vi "Main_control_cRIO.vi"() -> ()   [LabVIEW 2022 SP3]
uses:
  <vilib>/Platform/TimedLoop/XDataNode/timing_clust.ctl
  <vilib>/Platform/TimedLoop/XDataNode/nitl_modes.ctl
  <vilib>/Platform/TimedLoop/XDataNode/wakeup.ctl
  <vilib>/Analysis/baseanly.llb/Mean (DBL).vi
  a7aeaaac-04ba-4589-9d9a-9c348744fe2e.vi
  <vilib>/FPGAPlugInAG/cRIO-9045/niLvFpga_Open_cRIO-9045.vi
  <vilib>/rvi/interface/common/dynamic/niFpgaDynamicAddResources.vi
  <vilib>/Modbus/slave/Create Slave Instance (TCP).vi
  <vilib>/Utility/error.llb/Error Cluster From Error Code.vi
  <vilib>/rvi/errors/niLvFpgaAdjustHostInterfaceError.vi
  <vilib>/FPGAPlugInAG/Dynamic/niLvFpga_Close_Dynamic.vi
  <vilib>/rvi/interface/nirviOpenFPGA/nirviOpenFPGA.xnode
  FPGA Bitfiles/crio_FPGATarget_FPGAcomp_QzR2OHjg63E.lvbitx
  FPGA_1.vi
  <vilib>/platform/TimedLoop/XDataNode/XDataNode.xnode
  <vilib>/Comparison/Less/Less Functor/Less Functor.lvclass
  <vilib>/rvi/interface/nirviReadWriteControl/nirviReadWriteControl.xnode
  <vilib>/rvi/interface/nirviCloseFPGA/nirviCloseFPGA.xnode
  <vilib>/Modbus/slave/Modbus Slave.lvclass
  <vilib>/Modbus/master/Modbus Master.lvclass
  <vilib>/Platform/TimedLoop/XDataNode/XDNodeRunTimeDep.lvlib
  SubVIs/DAQ/DAQ_Termopares.lvlib
  SubVIs/CC Modbus/CC_Library.lvlib
  <vilib>/Analysis/NI_AALBase.lvlib
  <vilib>/rvi/interface/Simulation/niFpgaSimulationCallBeginRW.vi
  NiFpgaLv.dll
  <vilib>/ptbypt/NI_PtbyPt.lvlib
panel:
  out "isCamChangingSet?":bool
  out "PID 6":u32
  out "PID 2":u32
  out "PID 4":u32
  out "PID 8":u32
  out "PID 7":u32
  out "PID 5":u32
  out "PID 1":u32
  out "PID 3":u32
  out "W1.13":bool
  out "1.15":bool
  out "W1.7":bool
  out "W1.9":bool
  out "W1.11":bool
  out "W1.5":bool
  out "W1.3":bool
  out "W1.1":bool
  out "Segmento act":u16
  in  "reset warnings":bool
  out "Warnings table out":T1(array[cluster]) {"Time Stamp" format="%<%.3X %x>T"}
  in  "Activar Sim Bitron":bool
  out "LEL":bool
  out "CO":bool
  out "O2":bool
  out "LEL (%)":dbl
  out "CO (%)":dbl
  out "O2 (%)":dbl
  out "Array Warnings":bool[](array[boolean])
  out "Guardando resumen":bool=TRUE
  out "path":path
  out "T estabilidad calor":u32
  out "T transitorio calor":u32
  out "T estabilidad frio":u32
  out "T transitorio frio":u32
  out "Timer 4 (Inicio Estabilidad Calor)":u32
  out "Timer 3 (Inicio Transitorio Calor)":u32
  in  "Configuración":T2(tab)
  in  "Setpoint calor cam":dbl=55.0
  in  "Setpoints peltiers":dbl=85.0
  in  "Setpoint calor corte rampa":dbl=51.0
  in  "Setpoint Frío":dbl=-40.0 min=-28.0 max=70.0 step=0.1
  in  "Setpoint Corte Frío":dbl=-30.0 min=-28.0 max=70.0 step=0.1
  in  "Tiempò en estabilidad de Frío":u32=15
  in  "Tiempo minimo de ciclo":u32=70
  in  "Tiempo maximo de ciclo":u32=90
  in  "Cam ºC/min":dbl=2.2
  in  "Pelt ºC/min":dbl=2.5
  in  "T cliclo (Bitron FSM Sim)":u32
  in  "FSM Bitron Simulacion":i32
  in  "EnablePIs":bool[](array[boolean])=[FALSE, FALSE, FALSE, TRUE, FALSE, TRUE, FALSE, FALSE]
  in  "descarte media":i32=1
  out "DO H2 LAB":bool
  out "Array":dbl[][](array[numeric])
  out "error out":errorcluster
  in  "Enable Test PID":bool
  in  "Disable PID":bool
  in  "Test PID":u32[](array[numeric])
  out "PWM array":u32[](array[numeric])
  out "T_valves":dbl[](array[numeric]) format="%0.2f"
  out "PWM 8 (%)":u32
  out "PWM 7 (%)":u32
  out "PWM 6 (%)":u32
  out "PWM 5 (%)":u32
  out "PWM 4 (%)":u32
  out "PWM 3 (%)":u32=50 max=100
  out "SGL values":dbl[](array[numeric])
  out "Int values":u16[](array[numeric])
  out "Guardando en disco":bool
  out "array w/ subset deleted":dbl[][](array[numeric])
  out "Guardar Array":dbl[][](array[numeric])
  out "size(s)":i32
  out "TCP Connection Count":u32
  out "mean_T_valves":dbl format="%0.2f"
  out "Holding registers":u16[](array[numeric])
  out "First Time":bool=TRUE
  out "Timer 1 (Inicio transitorio frio)":u32
  out "Timer 2 (Inicio Estabilidad Frio)":u32
  in  "Rampa_cam":bool
  out "Temp_valves":dbl[](array[numeric]) format="%0.2f"
  in  "Rampa_pelt":bool
  in  "Minutos de medio ciclo":dbl=70.0
  out "Minutos":dbl
  out "Ciclos Totales":dbl
  out "segundos":dbl
  out "días":dbl
  out "Horas":dbl
  out "Minutos Totales":dbl
  out "t ensayo (s)":u64
  in  "Reset tempo":bool
  out "Iteration Duration":i64
  in  "Desconex_Control_Hum":bool
  out "PWM 2 (%)":u32
  out "Program running":bool
  in  "Pausa entrar":bool
  in  "Segmento":u16
  in  "Pausa":bool
  in  "stop Control General":bool
  in  "Run Program":bool
  in  "Entrada digital Bitron":bool
  in  "Cam_Hum_write":dbl min=0.0 max=100.0 step=0.1
  in  "Cam_Write_Set_Hum":bool
  in  "Cam_Temp_write":dbl min=-28.0 max=70.0 step=0.1
  in  "Cam_Write_Set_Temp":bool
  out "Cam_Temp_read":dbl min=-28.0 max=70.0 step=0.1
  out "Cam_Hum_read":dbl min=-28.0 max=70.0 step=0.1
  in  "Setpoint Peltiers":dbl=25.0
  in  "enable_PI":bool
  out "PWM 1 (%)":u32=50 max=100
  in  "STOP ALL":bool
  # "Temporizadores de ciclo"
  # "PID1 TEST"
  # "PID2 TEST"
  # "PID3 TEST"
  # "PID4 TEST"
  # "PID5 TEST"
  # "PID6 TEST"
  # "PID7 TEST"
  # "PID8 TEST"
  # "Peltiers"
  # "Cámara climática"
  # "min"
  # "min"
  # "min"
  # "min"
  # "segmento"
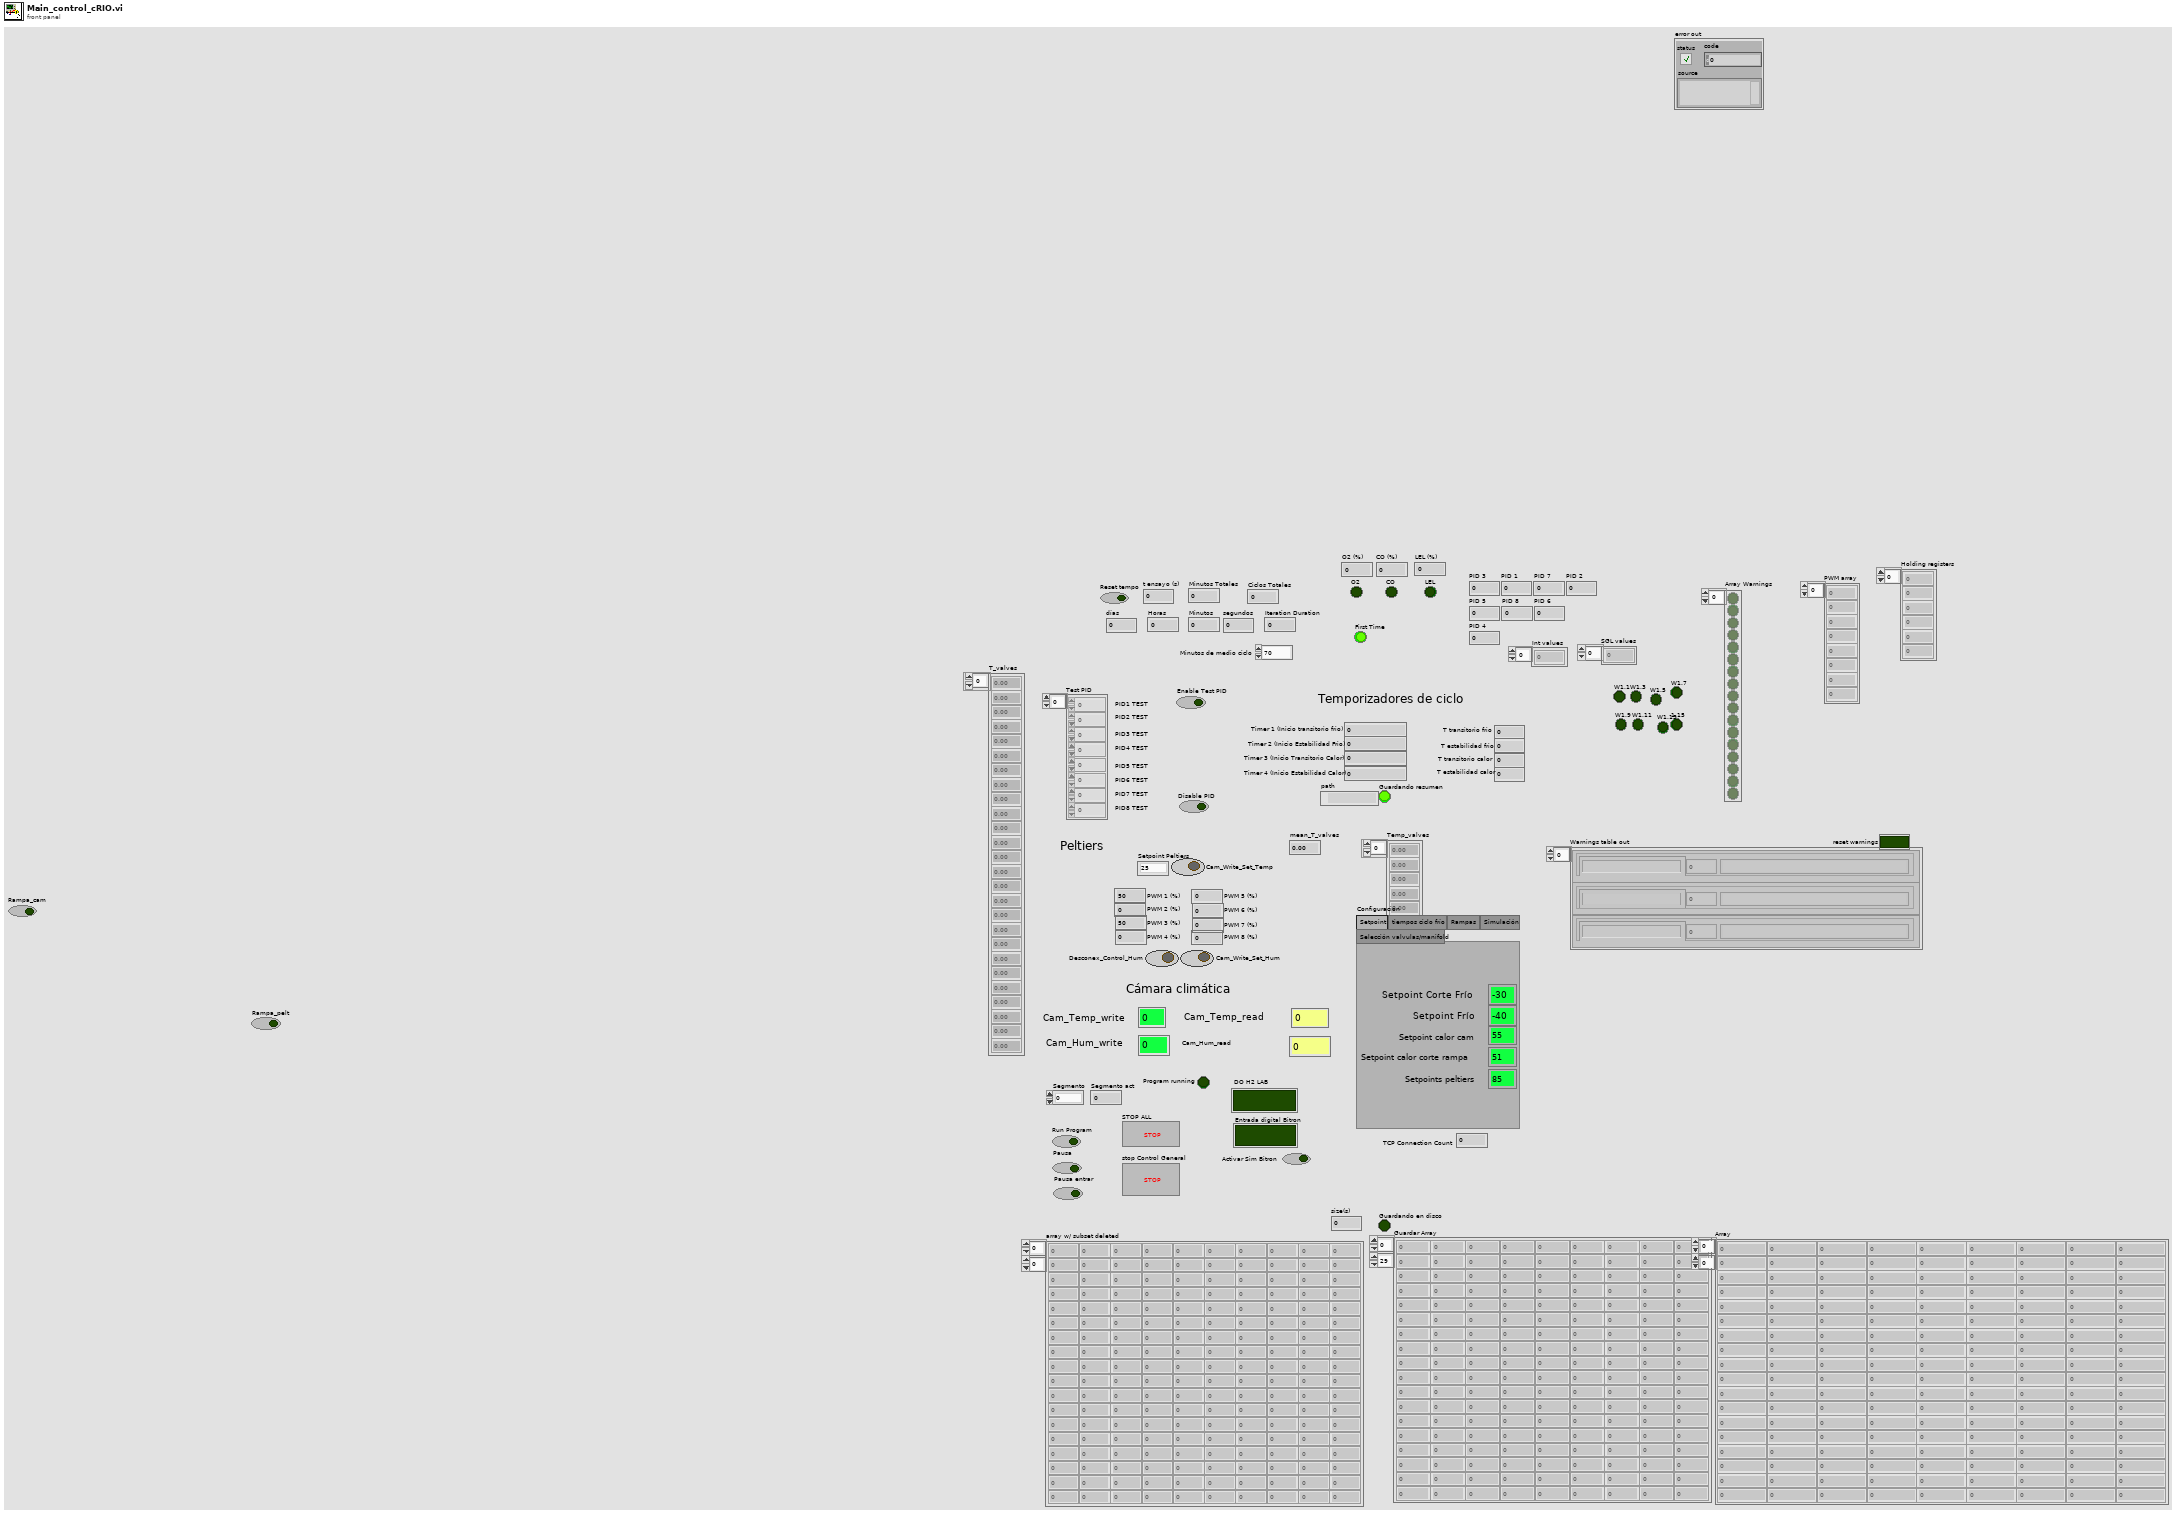
[diagram p1: front panel]
types:
  T1 = cluster{"Time Stamp":timestamp, "Descripcion":string, "Numeric":i32}[]
  T2 = enum32{"Setpoint", "tiempos ciclo frío", "Rampas ", "Simulación", "Selección valvulas/manifold"}
  T3 = enum8{"Enabled", "Disabled", "Disabled and Grayed Out"}
  T4 = typedef "XDNodeRunTimeDep.lvlib/timing_clust.ctl" = cluster{"Expected End [f-1]":u64, "Actual End [f-1]":u64, "Finished Late? [f-1]":bool, "Expected End [i-1]":u64, "Actual End [i-1]":u64, "Finished Late? [i-1]":bool, "Expected Start [i]":u64, "Actual Start [i]":u64, "Expected Start [f]":u64, "Actual Start [f]":u64, "Source Name":string, "Structure Name":string, "Period":i64, "Deadline":i64, "Offset":i64, "Start":i64, "Priority":i32, "Timeout":i32, "Mode":T5, "Wakeup Reason":T6, "Error":errorcluster, "Source Type":string, "Secondary Source Type":string, "Global End Time":u64, "Global Start Time":u64, "Frame Duration":u64, "Iteration Duration":u64, "Assigned CPU":i32, "I/O Scan Engine Mode":u32}
  T5 = typedef "XDNodeRunTimeDep.lvlib/nitl_modes.ctl" = enum32{"No Change", "Process missed periods, maintain original phase", "Discard missed periods, maintain original phase", "Process missed periods, ignore original phase", "Discard missed periods, ignore original phase"}
  T6 = typedef "XDNodeRunTimeDep.lvlib/wakeup.ctl" = enum32{"Normal", "Aborted", "Asynchronous wakeup", "Timing source error", "Timed loop error", "Timeout"}
  T7 = enum16{"open", "open or create", "create or replace", "create", "open (read-only)"}
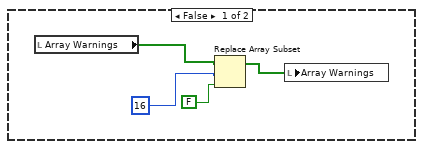
[diagram p3: hidden frame]
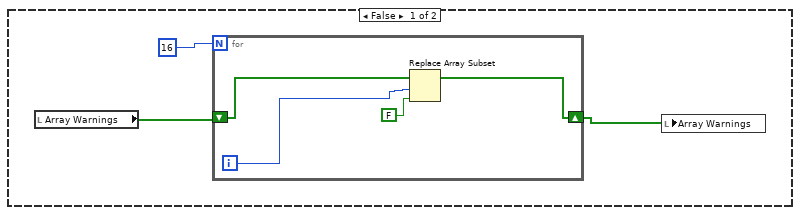
[diagram p4: hidden frame]
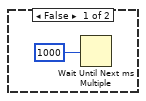
[diagram p7: hidden frame]
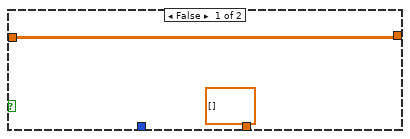
[diagram p8: hidden frame]
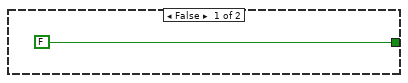
[diagram p9: hidden frame]
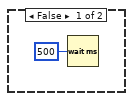
[diagram p14: hidden frame]
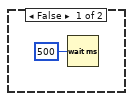
[diagram p15: hidden frame]
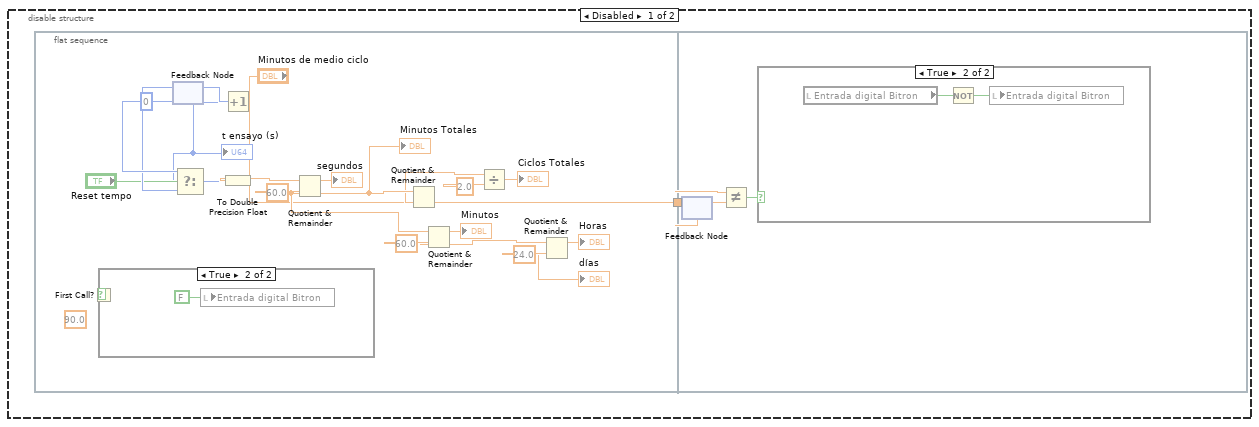
[diagram p17: hidden frame]
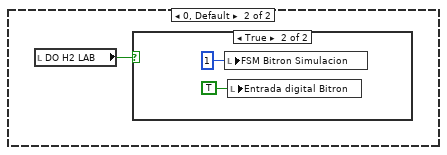
[diagram p20: hidden frame]
diagram:
  n1 = flat-sequence {
    tunnel: [w20] -> w16
    tunnel: [w19] -> w13
    tunnel: [w24] -> w12
    tunnel: [w29] -> w9
    tunnel: [w28] -> w8
    tunnel: [w22] -> w5
    tunnel: [w21] -> w4
    tunnel: [w17] -> w1
    tunnel: w16 -> [w61]
    tunnel: [w60] -> w15
    tunnel: [w59] -> w14
    tunnel: w13 -> [w58]
    tunnel: w12 -> [_]
    tunnel: [w51] -> w11
    tunnel: [w50] -> w10
    tunnel: w9 -> [w47]
    tunnel: w8 -> [w46]
    tunnel: [w45] -> w7
    tunnel: [w44] -> w6
    tunnel: w5 -> [_]
    tunnel: w4 -> [_]
    tunnel: [w32] -> w3
    tunnel: [w33] -> w2
    tunnel: w1 -> [_]
    tunnel: w15 -> [w1037]
    tunnel: w14 -> [w1036]
    tunnel: w11 -> [w1045]
    tunnel: w10 -> [w1044]
    tunnel: w7 -> [w1040]
    tunnel: w6 -> [w1039]
    tunnel: w3 -> [w1031]
    tunnel: w2 -> [w1032]
    frame #0 {
      w17 = FALSE ("Visible")
      w21 = bool[] [FALSE, FALSE, FALSE, FALSE, FALSE, FALSE, FALSE, FALSE, FALSE, FALSE, FALSE, FALSE, FALSE, FALSE, FALSE, FALSE, FALSE, FALSE, FALSE] ("Array Warnings")
      w22 = FALSE ("DO H2 LAB")
      w18 = u32 0 ("PWM 1 (%)")
      w26 = TRUE ("Visible")
      w30 = 10086 items=["J"=10072, "K"=10073, "N"=10077, "R"=10082, "S"=10085, "T"=10086, "B"=10047, "E"=10055] ("thermocouple type")
      w24 = FALSE ("Visible")
      n2 = local write "Entrada digital Bitron"(FALSE ("Entrada digital Bitron")) -> ()
      n3 = call "DAQ_connect.vi"("thermocouple type"=w30, "Array"=tag[] ["Mod2/ai0", "Mod2/ai1", "Mod2/ai2", "Mod2/ai3", "Mod2/ai4", "Mod2/ai5", "Mod2/ai6", "Mod2/ai7", "Mod2/ai8", "Mod2/ai9", "Mod2/ai10", "Mod2/ai11", "Mod2/ai12", "Mod2/ai13", "Mod2/ai14", "Mod2/ai15"]) -> ("error out"=w28:errorcluster, "Refnum out"=w29:refnum<k21>)  [unwired: 8 in]
      "error out" <- w28
      n4 = xnode "Open FPGA VI Reference"() -> ("FPGA VI Reference Out"=w20:refnum<k20>, "error out"=w19:errorcluster)  [unwired: 2 in]
      n5 = property on="Cam_Write_Set_Temp" class="Bool (strict)"("Visible"=w26) -> ()  [unwired: 2 in, 2 out]
      n6 = local write "PWM 8 (%)"(w18) -> ()
      n7 = property on="Cam_Write_Set_Hum" class="Bool (strict)"("Visible"=w26) -> ()  [unwired: 2 in, 2 out]
      n8 = local write "PWM 6 (%)"(w18) -> ()
      n9 = local write "PWM 7 (%)"(w18) -> ()
      n10 = local write "PWM 5 (%)"(w18) -> ()
      n11 = local write "PWM 4 (%)"(w18) -> ()
      n12 = local write "PWM 1 (%)"(w18) -> ()
      n13 = local write "PWM 2 (%)"(w18) -> ()
      n14 = local write "Rampa_pelt"(w24) -> ()
      n15 = local write "PWM 3 (%)"(w18) -> ()
      n16 = property on="enable_PI" class="Bool (strict)"("Visible"=w24) -> ()  [unwired: 2 in, 2 out]
      n17 = property on="Disable PID" class="Bool (strict)"("DisabledEnum"=T3."Disabled" ("Disabled")) -> ()  [unwired: 2 in, 2 out]
      n18 = local write "PID 8"(w18) -> ()
      n19 = local write "PID 7"(w18) -> ()
      n20 = local write "PID 6"(w18) -> ()
      n21 = local write "PID 5"(w18) -> ()
      n22 = local write "PID 1"(w18) -> ()
      n23 = local write "PID 2"(w18) -> ()
      n24 = local write "PID 4"(w18) -> ()
      n25 = local write "PID 3"(w18) -> ()
      n26 = property on="isCamChangingSet?" class="Bool (strict)"("Visible"=w17) -> ()  [unwired: 2 in, 2 out]
      "DO H2 LAB" <- w22
      "Array Warnings" <- w21
    }
    frame #1 {
      # "Running"
      n27 = node-c288() -> (w39:T4)  [unwired: 4 in]
      n28 = call "Nanodac_connect.vi"() -> ("error out"=w34:errorcluster, "Modbus Master out"=w35:refnum<class "Modbus Master.lvclass">)  [unwired: 10 in]
      n29 = node-c288() -> (w37:T4)  [unwired: 4 in]
      n30 = while "Adquisicion Resumen Datos/ciclo" {
        stop <- w237 stop-if-true
        w238 = FALSE ("Guardando resumen")
        # "CUIDADO! Al volver a empezar el ciclo, el Timer 1 va a ser el del siguiente ciclo, no el del que queremos registrar"
        # "0 -> First Time. Frío hasta -30 y señal bitron\n1 -> Transitorio frio\n2 -> Estabilidad frio\n3 -> Transitorio calor\n4 -> Estabilidad calor"
        # "Datos a guardar por ciclo:\n- Tiempo semiciclo frio\n- Tiempo estabilidad frio\n- Tiempo semiciclo calor\n- Tiempo estabilidad calor"
        n31 = local read "Segmento"() -> (w249:u16)
        n32 = feedback-in #1(w249) -> ()
        n33 = feedback #1(w249) -> (w248:u16)
        n34 = Equal?(x=w249, y=u16 1) -> (x = y?=w246:bool)
        n35 = local read "Program running"() -> (w235:bool)
        n36 = local write "Guardando resumen"(w238) -> ()
        n37 = local read "Segmento"() -> (w240:u16)
        n38 = Not Equal?(x=w248, y=u16 1) -> (x != y?=w245:bool)
        n39 = And(x=w246, y=w245) -> (x .and. y?=w236:bool)
        n40 = And(x=w235, y=w236) -> (x .and. y?=w234:bool)
        n41 = feedback #2(w240) -> (w241:u16)
        n42 = feedback-in #2(w240) -> ()
        n43 = Equal?(x=w240, y=u16 4) -> (x = y?=w243:bool)
        n44 = local read "Program running"() -> (w231:bool)
        n45 = case shown="True" w234 {
          tunnel: w238 -> [_ _]
          frame False {
          }
          frame True {
            n46 = flat-sequence {
              frame #0 {
                n47 = local read "Timer 4 (Inicio Estabilidad Calor)"() -> (w255:u32)
                n48 = local read "Timer 3 (Inicio Transitorio Calor)"() -> (w257:u32)
                n49 = local read "Timer 2 (Inicio Estabilidad Frio)"() -> (w258:u32)
                n50 = local read "Timer 1 (Inicio transitorio frio)"() -> (w256:u32)
                n51 = Subtract(x=w256, y=w255) -> (x-y=→"T estabilidad calor":u32)
                n52 = Subtract(x=w255, y=w257) -> (x-y=→"T transitorio calor":u32)
                n53 = Subtract(x=w257, y=w258) -> (x-y=→"T estabilidad frio":u32)
              }
              frame #1 {
                n54 = while {
                  stop <- w262 stop-if-true
                  n55 = local read "Guardando en disco"() -> (w263:bool)
                  n56 = Not(x=w263) -> (.not. x?=w262:bool)
                  n57 = Wait (ms)(milliseconds to wait=u32 500) -> ()  [unwired: 1 out]
                }
              }
              frame #2 {
                n58 = local read "T estabilidad calor"() -> (w268:u32)
                n59 = local read "T transitorio calor"() -> (w269:u32)
                n60 = local read "T estabilidad frio"() -> (w270:u32)
                n61 = local read "T transitorio frio"() -> (w271:u32)
                n62 = local read "path"() -> (w266:path)
                n63 = TDMS Open(10:T7."open or create" ("operation (0:open)"), 11:w266) -> (0:w276:errorcluster, 3:w277:refnum<k34>)  [unwired: 5 in]
                n64 = Build Array(w271, w270, w269, w268) -> (w267:u32[])
                n65 = TDMS Write(0:w277, 5:"Resumen Ciclos" ("group name in (Untitled)"), 7:string[] ["Time Transitorio frio (s)", "Time estabilidad frio (s)", "Time Transitorio calor (s)", "Time estabilidad calor (s)"] ("channel name(s) in (Untitled)"), 9:w267, 11:w276) -> (4:w275:refnum<k34>, 15:w274:errorcluster)  [unwired: 1 in, 2 out]
                n66 = TDMS Close(8:w274, 11:w275) -> ()  [unwired: 2 out]
                "Guardando resumen" <- TRUE
              }
            }
          }
        }
        n67 = Not Equal?(x=w241, y=u16 4) -> (x != y?=w244:bool)
        n68 = And(x=w243, y=w244) -> (x .and. y?=w233:bool)
        n69 = And(x=w233, y=w231) -> (x .and. y?=w232:bool)
        n70 = case shown="True" w232 {
          frame False {
          }
          frame True {
            n71 = local read "Timer 1 (Inicio transitorio frio)"() -> (w252:u32)
            n72 = local read "Timer 2 (Inicio Estabilidad Frio)"() -> (w251:u32)
            n73 = Subtract(x=w251, y=w252) -> (x-y=→"T transitorio frio":u32)
          }
        }
        n74 = local read "STOP ALL"() -> (w237:bool)
        n75 = Wait (ms)(milliseconds to wait=u32 500) -> ()  [unwired: 1 out]
      }
      n76 = timed-loop "Rampa SP Camara" {
        timing: w39 -> [_]
        timing-out: [_] -> w38
        stop <- w592 stop-if-true
        n77 = node-c288() -> ()  [unwired: 1 in, 1 out]
        n78 = case shown="True" "Rampa_cam" {
          frame False {
            n79 = Wait (ms)(milliseconds to wait=u32 500) -> ()  [unwired: 1 out]
          }
          frame True {
            n80 = flat-sequence {
              tunnel: [w602] -> w594
              tunnel: w594 -> [w617]
              frame #0 {
                # "10*1/3*10^-4 ºC cada 20ms"
                n81 = local read "Cam_Temp_write"() -> (w608:dbl)
                n82 = local read "Temp_valves"() -> (w600:dbl[])
                n83 = Divide(x=1.0, y=3.0) -> (x/y=w614:dbl)
                n84 = Multiply(x="Cam ºC/min", y=w614) -> (x*y=w612:dbl)
                n85 = Index Array(array=w600, index #1=0 ("index"), index #2=1 ("index")) -> (element #1=w597:dbl, element #2=w596:dbl)
                n86 = Divide(x=w612, y=1000.0) -> (x/y=w613:dbl)
                n87 = Add(x=w608, y=w613) -> (x+y=w610:dbl)
                n88 = Build Array(w597, w596) -> (w595:dbl[])
                n89 = call-poly <vilib>:"Mean.vi"("X"=w595) -> ("mean"=w601:dbl)  [unwired: 1 out]
                n90 = Greater Or Equal?(x=w610, y="Setpoint calor cam") -> (x >= y?=w603:bool)
                n91 = Greater Or Equal?(x=w601, y="Setpoint calor corte rampa") -> (x >= y?=w604:bool)
                n92 = Or(x=w603, y=w604) -> (x .or. y?=w602:bool)
                n93 = Select(t="Setpoint calor cam", s=w602, f=w610) -> (s? t:f=w609:dbl)
                n94 = local write "Cam_Temp_write"(w609) -> ()
              }
              frame #1 {
                n95 = Not(x=w617) -> (.not. x?=w618:bool)
                n96 = local write "Rampa_cam"(w618) -> ()
              }
            }
          }
        }
        n97 = local read "STOP ALL"() -> (w592:bool)
        n98 = node-c288() -> ()  [unwired: 1 in, 1 out]
      }
      n99 = node-c288() -> (w63:T4)  [unwired: 4 in]
      n100 = timed-loop "Warnings/Errores" {
        timing: w37 -> [_]
        timing-out: [_] -> w36
        shift-right: [w78] -> _
        shift-left: T1 [] ("Warnings table out") -> [w79]
        stop <- w81 stop-if-true
        n101 = node-c288() -> ()  [unwired: 1 in, 1 out]
        n102 = local read "Program running"() -> (w84:bool)
        n103 = local read "Pausa"() -> (w85:bool)
        n104 = Not(x=w85) -> (.not. x?=w83:bool)
        n105 = And(x=w84, y=w83) -> (x .and. y?=w82:bool)
        n106 = case shown="True" w82 {
          frame False {
          }
          frame True {
            # "0 -> First Time. Frío hasta -30 y señal bitron\n1 -> Transitorio frio\n2 -> Estabilidad frio\n3 -> Transitorio calor\n4 -> Estabilidad calor"
            # "Si estamos en semiciclo de calor\ny no hay pausa"
            n107 = local read "Segmento"() -> (w137:u16)
            n108 = Tick Count (ms)() -> (millisecond timer value=w131:u32)
            n109 = local read "LEL (%)"() -> (w124:dbl)
            n110 = feedback-in #3(w131) -> ()
            n111 = feedback #3(w131) -> (w130:u32)
            n112 = local read "Array Warnings"() -> (w120:bool[])
            n113 = local read "isCamChangingSet?"() -> (w89:bool)
            n114 = Equal?(x=w137, y=u16 3) -> (x = y?=w134:bool)
            n115 = Equal?(x=w137, y=u16 4) -> (x = y?=w133:bool)
            n116 = Subtract(x=w131, y=w130) -> (x-y=w129:u32)
            n117 = Greater?(x=w124, y=3.0) -> (0:w118:bool)
            n118 = Or(x=w134, y=w133) -> (x .or. y?=w132:bool)
            n119 = Replace Array Subset(array=w120, new element=w118, index=17) -> (w117:bool[])
            n120 = Select(t=u32 1000, s=w89, f=u32 60000 ("y")) -> (s? t:f=w86:u32)
            n121 = Greater Or Equal?(x=w129, y=w86) -> (x >= y?=w128:bool)
            n122 = Array Subset(array=w117, index=0, length=19) -> (w110:bool[])
            n123 = case shown="True" w132 {
              frame False {
                n124 = local read "Array Warnings"() -> (w169:bool[])
                n125 = for {
                  N: 16 -> [_]
                  shift-right: [w171] -> w168
                  shift-left: w169 -> [w172]
                  i -> [w174]
                  n126 = Replace Array Subset(array=w172, new element=FALSE ("new element/subarray"), index=w174) -> (w171:bool[])
                }
                n127 = local write "Array Warnings"(w168) -> ()
              }
              frame True {
                n128 = local read "Setpoint Peltiers"() -> (w215:dbl)
                n129 = local read "T_valves"() -> (w214:dbl[])
                n130 = for {
                  N: 16 -> [_]
                  tunnel: w215 -> [w222]
                  tunnel: w214 -> [w220]
                  shift-right: [w216] -> w195
                  shift-left: bool[] [FALSE, FALSE, FALSE, FALSE, FALSE, FALSE, FALSE, FALSE, FALSE, FALSE, FALSE, FALSE, FALSE, FALSE, FALSE, FALSE] -> [w217]
                  i -> [w219]
                  n131 = Index Array(array=w220, index=w219) -> (element=w218:dbl)
                  n132 = Subtract(x=w222, y=w218) -> (x-y=w225:dbl)
                  n133 = Absolute Value(x=w225) -> (abs(x)=w224:dbl)
                  n134 = Greater?(x=w224, y=20.0) -> (0:w221:bool)
                  n135 = Replace Array Subset(array=w217, new element=w221, index=w219) -> (w216:bool[])
                }
                n136 = local read "Array Warnings"() -> (w194:bool[])
                n137 = Index Array(array=w195, index #1=0 ("index"), index #2=2 ("index"), index #3=4 ("index"), index #4=6 ("index"), index #5=8 ("index"), index #6=10 ("index"), index #7=12 ("index"), index #8=14 ("index"), index #9=1 ("index"), index #10=3 ("index"), index #11=5 ("index"), index #12=7 ("index"), index #13=9 ("index"), index #14=11 ("index"), index #15=13 ("index"), index #16=15 ("index")) -> (element #1=w211:bool, element #2=w210:bool, element #3=w209:bool, element #4=w208:bool, element #5=w207:bool, element #6=w206:bool, element #7=w205:bool, element #8=w204:bool, element #9=w203:bool, element #10=w202:bool, element #11=w201:bool, element #12=w200:bool, element #13=w199:bool, element #14=w198:bool, element #15=w197:bool, element #16=w196:bool)
                n138 = Build Array(w211, w210, w209, w208, w207, w206, w205, w204, w203, w202, w201, w200, w199, w198, w197, w196) -> (w192:bool[])
                n139 = Replace Array Subset(array=w194, new element=w192, index=0) -> (w191:bool[])
                n140 = local write "Array Warnings"(w191) -> ()
              }
            }
            n141 = case shown="True" w128 {
              tunnel: w129 -> [_ w164]
              frame False {
                n142 = local read "Array Warnings"() -> (w141:bool[])
                n143 = Replace Array Subset(array=w141, new element=FALSE ("new element/subarray"), index=16) -> (w138:bool[])
                n144 = local write "Array Warnings"(w138) -> ()
              }
              frame True {
                n145 = local read "Cam_Temp_write"() -> (w155:dbl)
                n146 = local read "Cam_Temp_read"() -> (w153:dbl)
                n147 = Subtract(x=w153, y=w155) -> (x-y=w167:dbl)
                n148 = feedback #4(w153) -> (w154:dbl)
                n149 = feedback-in #4(w153) -> ()
                n150 = Absolute Value(x=w167) -> (abs(x)=w145:dbl)
                n151 = Subtract(x=w153, y=w154) -> (x-y=w165:dbl)
                n152 = Greater Or Equal?(x=w145, y=3.0) -> (x >= y?=w144:bool)
                n153 = Absolute Value(x=w165) -> (abs(x)=w161:dbl)
                n154 = Divide(x=w164, y=u32 60000) -> (x/y=w162:dbl)
                n155 = Divide(x=w161, y=w162) -> (x/y=w148:dbl)
                n156 = call <vilib>:"Mean PtByPt.vi"("x"=w148) -> ("mean"=w147:dbl)  [unwired: 3 in, 1 out]
                n157 = feedback-in #5(w145) -> ()
                n158 = feedback #5(w145) -> (w146:dbl)
                n159 = Not Equal To 0?(x=w146) -> (x != 0?=w142:bool)
                "isCamChangingSet?" <- w142
                n160 = Less?(x=w147, y=0.2) -> (x < y?=w159:bool)
                n161 = And(x=w142, y=w144) -> (x .and. y?=w143:bool)
                n162 = local read "Array Warnings"() -> (w150:bool[])
                n163 = First Call?() -> (First Call?: T/F=w156:bool)
                n164 = And(x=w143, y=w159) -> (x .and. y?=w158:bool)
                n165 = Not(x=w156) -> (.not. x?=w157:bool)
                n166 = And(x=w157, y=w158) -> (x .and. y?=w149:bool)
                n167 = Replace Array Subset(array=w150, new element=w149, index=16) -> (w152:bool[])
                n168 = local write "Array Warnings"(w152) -> ()
              }
            }
            n169 = local write "Array Warnings"(w110) -> ()
            n170 = local read "O2 (%)"() -> (w109:dbl)
            n171 = local read "Array Warnings"() -> (w123:bool[])
            n172 = Greater?(x=w109, y=25.0) -> (0:w125:bool)
            n173 = Less?(x=w109, y=10.0) -> (x < y?=w107:bool)
            n174 = Or(x=w125, y=w107) -> (x .or. y?=w121:bool)
            n175 = Replace Array Subset(array=w123, new element=w121, index=18) -> (w112:bool[])
            n176 = Array Subset(array=w112, index=0, length=19) -> (w111:bool[])
            n177 = local write "Array Warnings"(w111) -> ()
            n178 = local read "Array Warnings"() -> (w106:bool[])
            n179 = Index Array(array=w106, index #1=0 ("index"), index #2=2 ("index"), index #3=4 ("index"), index #4=6 ("index"), index #5=8 ("index"), index #6=10 ("index"), index #7=12 ("index"), index #8=14 ("index")) -> (element #1=→"W1.1":bool, element #2=→"W1.3":bool, element #3=→"W1.5":bool, element #4=→"W1.7":bool, element #5=→"W1.9":bool, element #6=→"W1.11":bool, element #7=→"W1.13":bool, element #8=→"1.15":bool)
          }
        }
        n180 = local read "Array Warnings"() -> (w80:bool[])
        n181 = call "Historical Warnings (SubVI).vi"("Warnings bool array"=w80, "in"="reset warnings", "warnings table in"=w79) -> ("Warnings table out"=w78:T1)  [unwired: 8 in]
        "Warnings table out" <- w78
        n182 = local read "STOP ALL"() -> (w81:bool)
        n183 = node-c288() -> ()  [unwired: 1 in, 1 out]
      }
      n184 = while "MODBUS CC NANODAC" {
        tunnel: w35 -> [w76]
        tunnel: w34 -> [w75]
        tunnel: [w65] -> w33
        tunnel: [w64] -> w32
        stop <- w74 stop-if-true
        n185 = call "Nanodac_lectura.vi"("Modbus Master in"=w76, "error in (no error)"=w75) -> ("Modbus Master out"=w65:refnum<class "Modbus Master.lvclass">, 16:"O2, CO, LEL"=w72:dbl[], 17:"O2, CO, LEL"=w73:bool[], "error out"=w64:errorcluster)  [unwired: 14 in]
        n186 = Index Array(array=w73) -> (element #1=→"O2":bool, element #2=→"CO":bool, element #3=→"LEL":bool)  [unwired: 3 in]
        n187 = Index Array(array=w72) -> (element #1=→"O2 (%)":dbl, element #2=→"CO (%)":dbl, element #3=→"LEL (%)":dbl)  [unwired: 3 in]
        n188 = local read "STOP ALL"() -> (w74:bool)
      }
      n189 = while "Modbus Slave" {
        stop <- w405 stop-if-true
        n190 = call-poly <vilib>:"Create Slave Instance.vi"() -> ("error out"=w408:errorcluster, "TCP slave instance"=w409:refnum<class "Modbus Slave.lvclass">)  [unwired: 10 in]
        n191 = while {
          shift-right: [w421] -> w407
          shift-left: w409 -> [w423]
          shift-right: [w420] -> w406
          shift-left: w408 -> [w422]
          stop <- w415 stop-if-true
          n192 = property class="Modbus Slave"(reference=w423, error in=w422) -> (reference out=w421:refnum<class "Modbus Slave.lvclass">, error out=w420:errorcluster, "Data Access:TCP Connection Count"=w419:u32)
          "TCP Connection Count" <- w419
          n193 = Not Equal?(x=w419, y=u32 0) -> (x != y?=w417:bool)
          n194 = local read "STOP ALL"() -> (w416:bool)
          n195 = Or(x=w417, y=w416) -> (x .or. y?=w415:bool)
        }
        n196 = node-c288() -> (w414:T4)  [unwired: 4 in]
        n197 = timed-loop {
          timing: w414 -> [_]
          timing-out: [_] -> w413
          shift-right: [w488] -> w411
          shift-left: w407 -> [w499]
          shift-right: [w487] -> w410
          shift-left: w406 -> [w497]
          shift-right: [w490] -> _
          shift-left: u16[] [0, 0, 0, 0, 0, 0, 0, 0, 0, 0, 0, 0, 0, 0, 0, 0, 0, 0, 0, 0, 0, 0, 0, 0, 0, 0, 0, 0, 0, 0, 0, 0, 0, 0, 0, 0, 0, 0, 0, 0, 0, 0, 0, 0, 0] -> [w491]
          stop <- w483 stop-if-true
          # "Temp_BobV3-8"
          # "Temp_valves\nTemp_bobs"
          n198 = node-c288() -> ()  [unwired: 1 in, 1 out]
          n199 = local read "Entrada digital Bitron"() -> (w472:bool)
          n200 = local read "Array Warnings"() -> (w455:bool[])
          n201 = local read "Program running"() -> (w504:bool)
          n202 = local read "DO H2 LAB"() -> (w459:bool)
          n203 = local read "T_valves"() -> (w467:dbl[])
          n204 = local read "enable_PI"() -> (w503:bool)
          n205 = local read "Cam_Temp_write"() -> (w468:dbl)
          n206 = local read "Cam_Temp_read"() -> (w469:dbl)
          n207 = local read "Cam_Hum_read"() -> (w471:dbl)
          n208 = local read "Cam_Hum_write"() -> (w470:dbl)
          n209 = local read "mean_T_valves"() -> (w434:dbl)
          n210 = local read "Setpoint Peltiers"() -> (w502:dbl)
          n211 = Build Array (concatenate)(w504, w503, w472, w459, w455) -> (w498:bool[])
          n212 = Build Array(w471, w470, w469, w468, w434) -> (w465:dbl[])
          n213 = Build Array(w502) -> (w466:dbl[])
          n214 = local read "Segmento act"() -> (w501:u16)
          n215 = local read "PWM array"() -> (w461:u32[])
          n216 = Build Array (concatenate)(w466, w467, w465) -> (w464:dbl[])
          "SGL values" <- w464
          n217 = Array Size(array=w464) -> (size(s)=w492:i32)
          n218 = To Unsigned Word Integer(number=w461) -> (unsigned 16bit integer=w462:u16[])
          n219 = call-dynamic "Write Multiple Coils.vi"("error in (no error)"=w497, "coil values"=w498, "starting address"=u16 1, "Modbus slave in"=w499) -> ("error out"=w494:errorcluster, "Modbus slave out"=w495:refnum<class "Modbus Slave.lvclass">)  [unwired: 6 in]
          n220 = Build Array(w501) -> (w463:u16[])
          n221 = Build Array (concatenate)(w463, w462) -> (w460:u16[])
          "Int values" <- w460
          n222 = for {
            N: w492 -> [_]
            tunnel: w464 -> [w586] mode=indexing
            shift-right: [w577] -> w490
            shift-left: w491 -> [w578]
            i -> [w585]
            n223 = call "double_2u16.vi"("Entrada"=w586) -> ("Salida 2"=w582:u16, "Salida 1"=w583:u16)  [unwired: 9 in]
            n224 = Multiply(x=2, y=w585) -> (x*y=w581:i32)
            n225 = Add(x=1, y=w581) -> (x+y=w579:i32)
            n226 = Replace Array Subset(array=w578, new element #1=w583, index #1=w581, new element #2=w582, index #2=w579) -> (w577:u16[])
          }
          n227 = for {
            tunnel: w460 -> [w576] mode=indexing
            tunnel: [w574] -> w489 mode=indexing
            n228 = Add(x=w576, y=u16 10000) -> (x+y=w574:u16)
          }
          n229 = Build Array (concatenate)(w489, w490) -> (w493:u16[])
          "Holding registers" <- w493
          n230 = call-dynamic "Write Multiple Holding Registers.vi"("error in (no error)"=w494, "holding register values"=w493, "starting address"=u16 100, "Modbus slave in"=w495) -> ("error out"=w480:errorcluster, "Modbus slave out"=w481:refnum<class "Modbus Slave.lvclass">)  [unwired: 6 in]
          n231 = call-dynamic "Read Coils.vi"("error in (no error)"=w480, "number of coils"=u16 5, "starting address"=u16 200, "Modbus slave in"=w481) -> ("error out"=w457:errorcluster, "coil values"=w474:bool[], "Modbus slave out"=w458:refnum<class "Modbus Slave.lvclass">)  [unwired: 5 in]
          n232 = Index Array(array=w474) -> (element #1=w477:bool, element #2=w476:bool, element #3=w475:bool, element #4=w473:bool, element #5=w456:bool)  [unwired: 5 in]
          n233 = local write "Run Program"(w477) -> ()
          n234 = local write "Pausa"(w476) -> ()
          n235 = local write "Pausa entrar"(w475) -> ()
          n236 = local write "stop Control General"(w473) -> ()
          n237 = case shown="True" w456 {
            tunnel: [w532 w534] -> w433
            tunnel: w458 -> [w532 w542]
            tunnel: w457 -> [w531 w541]
            tunnel: [w531 w533] -> w432
            frame False {
            }
            frame True {
              w545 = u16 22 ("number of holding registers")
              n238 = call-dynamic "Read Coils.vi"("error in (no error)"=w541, "number of coils"=u16 1, "starting address"=u16 205, "Modbus slave in"=w542) -> ("error out"=w540:errorcluster, "coil values"=w535:bool[], "Modbus slave out"=w539:refnum<class "Modbus Slave.lvclass">)  [unwired: 5 in]
              n239 = Index Array(array=w535) -> (element=w536:bool)  [unwired: 1 in]
              n240 = local write "Activar Sim Bitron"(w536) -> ()
              n241 = Quotient & Remainder(x=w545, y=u16 2) -> (floor(x/y)=w543:u16)  [unwired: 1 out]
              n242 = call-dynamic "Read Holding Registers.vi"("error in (no error)"=w540, "number of holding registers"=w545, "starting address"=u16 300, "Modbus slave in"=w539) -> ("error out"=w533:errorcluster, "register values"=w558:u16[], "Modbus slave out"=w534:refnum<class "Modbus Slave.lvclass">)  [unwired: 5 in]
              n243 = for {
                N: w543 -> [_]
                tunnel: [w566] -> w557 mode=indexing
                tunnel: w558 -> [w562]
                i -> [w573]
                n244 = Multiply(x=2, y=w573) -> (x*y=w571:i32)
                n245 = Add(x=w571, y=1) -> (x+y=w569:i32)
                n246 = Index Array(array=w562, index #1=w571, index #2=w569) -> (element #1=w561:u16, element #2=w560:u16)
                n247 = Join Numbers(hi=w561, lo=w560) -> ((hi.lo)=w568:u32)
                n248 = To Single Precision Float(number=w568) -> (single precision float=w565:sgl)
                n249 = Subtract(x=w565, y=sgl 10000.0) -> (x-y=w563:sgl)
                n250 = Divide(x=w563, y=sgl 100.0) -> (x/y=w566:sgl)
              }
              n251 = Index Array(array=w557) -> (element #1=w556:sgl, element #2=w555:sgl, element #3=w554:sgl, element #4=w553:sgl, element #5=w552:sgl, element #6=w551:sgl, element #7=w550:sgl, element #8=w549:sgl, element #9=w548:sgl, element #10=w547:sgl, element #11=w546:sgl)  [unwired: 11 in]
              n252 = local write "Tiempò en estabilidad de Frío"(w551) -> ()
              n253 = local write "Setpoint calor corte rampa"(w553) -> ()
              n254 = local write "Tiempo maximo de ciclo"(w549) -> ()
              n255 = local write "Tiempo minimo de ciclo"(w550) -> ()
              n256 = local write "T cliclo (Bitron FSM Sim)"(w546) -> ()
              n257 = local write "Setpoint Corte Frío"(w556) -> ()
              n258 = local write "Setpoint calor cam"(w554) -> ()
              n259 = local write "Setpoints peltiers"(w552) -> ()
              n260 = local write "Setpoint Frío"(w555) -> ()
              n261 = local write "Cam ºC/min"(w548) -> ()
              n262 = local write "Pelt ºC/min"(w547) -> ()
            }
          }
          n263 = call-dynamic "Read Coils.vi"("error in (no error)"=w432, "number of coils"=u16 1, "starting address"=u16 400, "Modbus slave in"=w433) -> ("error out"=w428:errorcluster, "coil values"=w429:bool[], "Modbus slave out"=w427:refnum<class "Modbus Slave.lvclass">)  [unwired: 5 in]
          n264 = Index Array(array=w429) -> (element=w424:bool)  [unwired: 1 in]
          n265 = local write "Disable PID"(w424) -> ()
          n266 = case shown="True" w424 {
            tunnel: w428 -> [w505 w520]
            tunnel: w427 -> [w506 w521]
            tunnel: [w506 w508] -> w426
            tunnel: [w505 w507] -> w425
            frame False {
            }
            frame True {
              n267 = call-dynamic "Read Holding Registers.vi"("error in (no error)"=w520, "number of holding registers"=u16 8, "starting address"=u16 410, "Modbus slave in"=w521) -> ("error out"=w507:errorcluster, "register values"=w517:u16[], "Modbus slave out"=w508:refnum<class "Modbus Slave.lvclass">)  [unwired: 5 in]
              n268 = Index Array(array=w517) -> (element #1=w516:u16, element #2=w515:u16, element #3=w514:u16, element #4=w513:u16, element #5=w512:u16, element #6=w511:u16, element #7=w510:u16, element #8=w509:u16)  [unwired: 8 in]
              n269 = local write "PWM 4 (%)"(w513) -> ()
              n270 = local write "PWM 1 (%)"(w516) -> ()
              n271 = local write "PWM 2 (%)"(w515) -> ()
              n272 = local write "PWM 5 (%)"(w512) -> ()
              n273 = local write "PWM 6 (%)"(w511) -> ()
              n274 = local write "PWM 7 (%)"(w510) -> ()
              n275 = local write "PWM 8 (%)"(w509) -> ()
              n276 = local write "PWM 3 (%)"(w514) -> ()
            }
          }
          n277 = local read "STOP ALL"() -> (w482:bool)
          n278 = call-dynamic "Read Coils.vi"("error in (no error)"=w425, "number of coils"=u16 8, "starting address"=u16 240, "Modbus slave in"=w426) -> ("error out"=w435:errorcluster, "coil values"=w445:bool[], "Modbus slave out"=w436:refnum<class "Modbus Slave.lvclass">)  [unwired: 5 in]
          n279 = local write "EnablePIs"(w445) -> ()
          n280 = call-dynamic "Read Holding Registers.vi"("error in (no error)"=w435, "number of holding registers"=u16 1, "starting address"=u16 350, "Modbus slave in"=w436) -> ("error out"=w437:errorcluster, "register values"=w441:u16[], "Modbus slave out"=w438:refnum<class "Modbus Slave.lvclass">)  [unwired: 5 in]
          n281 = Index Array(array=w441) -> (element=w442:u16)  [unwired: 1 in]
          n282 = local write "descarte media"(w442) -> ()
          n283 = call-dynamic "Read Coils.vi"("error in (no error)"=w437, "number of coils"=u16 1, "starting address"=u16 250, "Modbus slave in"=w438) -> ("error out"=w451:errorcluster, "coil values"=w448:bool[], "Modbus slave out"=w452:refnum<class "Modbus Slave.lvclass">)  [unwired: 5 in]
          n284 = Index Array(array=w448, index=0) -> (element=w446:bool)
          n285 = local write "Enable Test PID"(w446) -> ()
          n286 = case shown="True" w446 {
            tunnel: [w523 w530] -> w454
            tunnel: [w522 w529] -> w453
            tunnel: w452 -> [w523 w528]
            tunnel: w451 -> [w522 w527]
            frame False {
            }
            frame True {
              n287 = call-dynamic "Read Holding Registers.vi"("error in (no error)"=w527, "number of holding registers"=u16 8, "starting address"=u16 260, "Modbus slave in"=w528) -> ("error out"=w529:errorcluster, "register values"=w524:u16[], "Modbus slave out"=w530:refnum<class "Modbus Slave.lvclass">)  [unwired: 5 in]
              n288 = local write "Test PID"(w524) -> ()
            }
          }
          n289 = property class="Modbus Slave"(reference=w454, error in=w453) -> (reference out=w488:refnum<class "Modbus Slave.lvclass">, error out=w487:errorcluster, "Data Access:TCP Connection Count"=w486:u32)
          n290 = Equal?(x=w486, y=u32 0) -> (x = y?=w484:bool)
          n291 = Or(x=w484, y=w482) -> (x .or. y?=w483:bool)
          n292 = node-c288() -> ()  [unwired: 1 in, 1 out]
        }
        n293 = node-c288(w413) -> ()  [unwired: 1 out]
        n294 = local read "STOP ALL"() -> (w405:bool)
        n295 = call-dynamic "Close.vi"("error in (no error)"=w410, "Modbus slave in"=w411) -> ()  [unwired: 9 in, 1 out]
      }
      n296 = timed-loop "FPGA Aquisicion y control" {
        timing: w63 -> [_]
        timing-out: [_] -> w62
        tunnel: w61 -> [w1016]
        tunnel: [w999] -> w60
        tunnel: [w1015] -> w59
        tunnel: w58 -> [w1014]
        tunnel: w47 -> [w1013]
        tunnel: w46 -> [w1012]
        tunnel: [w1011] -> w45
        tunnel: [w1010] -> w44
        stop <- "STOP ALL" stop-if-true
        # "1 y 1 de momento, cuando haya mas valvulas, 2 y 2"
        n297 = node-c288() -> ()  [unwired: 1 in, 1 out]
        n298 = local read "PWM 8 (%)"() -> (w1000:u32)
        n299 = local read "PWM 6 (%)"() -> (w1002:u32)
        n300 = local read "PWM 7 (%)"() -> (w1001:u32)
        n301 = local read "PWM 5 (%)"() -> (w1003:u32)
        n302 = local read "PWM 4 (%)"() -> (w1004:u32)
        n303 = local read "PWM 1 (%)"() -> (w1007:u32)
        n304 = local read "PWM 2 (%)"() -> (w1006:u32)
        n305 = local read "PWM 3 (%)"() -> (w1005:u32)
        n306 = xnode "Read/Write Control"("FPGA VI Reference In"=w1016, "error in"=w1014, "PWM_DO0"=w1007, "PWM_DO1"=w1006, "PWM_DO2"=w1005, "PWM_DO3"=w1004, "PWM_DO4"=w1003, "PWM_DO5"=w1002, "PWM_DO6"=w1001, "PWM_DO7"=w1000) -> ("FPGA VI Reference Out"=w999:refnum<k20>, "error out"=w1015:errorcluster)
        n307 = call "DAQ_read_T_dT.vi"("error in (no error)"=w1012, "Refnum in"=w1013) -> ("error out"=w1010:errorcluster, "data"=w986:dbl[], "Refnum out"=w1011:refnum<k21>)  [unwired: 7 in]
        "Temp_valves" <- w986
        "T_valves" <- w986
        n308 = Build Array(w1007, w1006, w1005, w1004, w1003, w1002, w1001, w1000) -> (→"PWM array":u32[])
        n309 = local read "EnablePIs"() -> (w998:bool[])
        n310 = Split 1D Array(array=w986, index=8) -> (second subarray=w996:dbl[])  [unwired: 1 out]
        n311 = for {
          tunnel: w998 -> [w1018] mode=indexing
          tunnel: w996 -> [w1021] mode=indexing
          shift-right: [w1019] -> w995
          shift-left: dbl[] [] -> [w1020]
          n312 = case shown="False" w1018 {
            tunnel: w1021 -> [_ w1025]
            tunnel: w1020 -> [w1022 w1024]
            tunnel: [w1022 w1023] -> w1019
            frame False {
            }
            frame True {
              n313 = Insert Into Array(array=w1024, new element=w1025) -> (w1023:dbl[])  [unwired: 1 in]
            }
          }
        }
        n314 = call "Sort 1D Array.vim"("unsorted array"=w995) -> ("sorted array"=w994:dbl[])  [unwired: 10 in]
        n315 = Array Size(array=w994) -> (size(s)=w993:i32)
        n316 = Multiply(x=2, y="descarte media") -> (x*y=w987:i32)
        n317 = Subtract(x=w993, y=w987) -> (x-y=w992:i32)
        n318 = Array Subset(array=w994, index="descarte media", length=w992) -> (w991:dbl[])
        n319 = call-poly <vilib>:"Mean.vi"("X"=w991) -> ("mean"=→"mean_T_valves":dbl)  [unwired: 1 out]
        n320 = node-c288() -> ()  [unwired: 1 in, 1 out]
      }
      n321 = node-c288(w38) -> ()  [unwired: 1 out]
      n322 = node-c288() -> (w41:T4)  [unwired: 4 in]
      n323 = timed-loop "Rampa SP Peltiers" {
        timing: w41 -> [_]
        timing-out: [_] -> w40
        stop <- w624 stop-if-true
        n324 = node-c288() -> ()  [unwired: 1 in, 1 out]
        n325 = case shown="True" "Rampa_pelt" {
          frame False {
            n326 = Wait (ms)(milliseconds to wait=u32 500) -> ()  [unwired: 1 out]
          }
          frame True {
            n327 = flat-sequence {
              tunnel: [w631] -> w626
              tunnel: w626 -> [w639]
              frame #0 {
                # "20*1/3*10^-4 ºC cada 20ms"
                n328 = local read "Setpoint Peltiers"() -> (w629:dbl)
                n329 = Divide(x=1.0, y=3.0) -> (x/y=w636:dbl)
                n330 = Multiply(x="Pelt ºC/min", y=w636) -> (x*y=w634:dbl)
                n331 = Divide(x=w634, y=1000.0) -> (x/y=w635:dbl)
                n332 = Add(x=w629, y=w635) -> (x+y=w632:dbl)
                n333 = Greater Or Equal?(x=w632, y="Setpoints peltiers") -> (x >= y?=w631:bool)
                n334 = Select(t="Setpoints peltiers", s=w631, f=w632) -> (s? t:f=w630:dbl)
                n335 = local write "Setpoint Peltiers"(w630) -> ()
              }
              frame #1 {
                n336 = Not(x=w639) -> (.not. x?=w640:bool)
                n337 = local write "Rampa_pelt"(w640) -> ()
              }
            }
          }
        }
        n338 = local read "STOP ALL"() -> (w624:bool)
        n339 = node-c288() -> ()  [unwired: 1 in, 1 out]
      }
      n340 = while "Guardado de Datos" {
        stop <- w279 stop-if-true
        n341 = local read "Program running"() -> (w278:bool)
        n342 = case shown="True" w278 {
          frame False {
            n343 = Wait Until Next ms Multiple(millisecond multiple=u32 1000 ("milliseconds to wait")) -> ()  [unwired: 1 out]
          }
          frame True {
            w289 = dbl[][] []
            n344 = Get Date/Time In Seconds() -> (seconds since 1Jan1904=w288:timestamp)
            n345 = Format Date/Time String(time format string (%c)="%Y_%m_%d_%H_%M", seconds (now)=w288) -> (date/time string=w284:string)  [unwired: 1 in]
            n346 = local write "array w/ subset deleted"(w289) -> ()
            n347 = local write "Guardar Array"(w289) -> ()
            n348 = Concatenate Strings("/media/sdb1/Datos_Bitron/" ("string"), w284, "_data CC.tdms" ("string")) -> (w285:string)
            n349 = String To Path(string=w285) -> (path=w282:path)
            "path" <- w282
            n350 = while {
              shift-right: [w336] -> _
              shift-left: w289 -> [w339]
              tunnel: w282 -> [w327]
              tunnel: [FALSE ("stop Control General")] -> w281
              i -> [w344]
              stop <- w310 stop-if-true
              # "10 minutos = 599"
              n351 = local read "Program running"() -> (w304:bool)
              n352 = local read "enable_PI"() -> (w303:bool)
              n353 = local read "Entrada digital Bitron"() -> (w302:bool)
              n354 = local read "Run Program"() -> (w301:bool)
              n355 = local read "Pausa"() -> (w300:bool)
              n356 = local read "Pausa entrar"() -> (w299:bool)
              n357 = local read "stop Control General"() -> (w298:bool)
              n358 = local read "DO H2 LAB"() -> (w295:bool)
              n359 = local read "TCP Connection Count"() -> (w316:u32)
              n360 = local read "SGL values"() -> (w325:dbl[])
              n361 = local read "Int values"() -> (w326:u16[])
              n362 = Tick Count (ms)() -> (millisecond timer value=w330:u32)
              n363 = To Double Precision Float(number=w326) -> (double precision float=w324:dbl[])
              n364 = To Double Precision Float(number=w325) -> (double precision float=w323:dbl[])
              n365 = Divide(x=w330, y=u32 1000) -> (x/y=w322:dbl)
              n366 = Greater?(x=w316, y=u32 0) -> (0:w314:bool)
              n367 = Boolean To (0,1)(Boolean=w314) -> (0, 1=w318:i16)
              n368 = To Double Precision Float(number=w318) -> (double precision float=w317:dbl)
              n369 = Build Array(w304, w303, w302, w301, w300, w299, w298, w295) -> (w297:bool[])
              n370 = Build Array(w317) -> (w296:dbl[])
              n371 = Boolean To (0,1)(Boolean=w297) -> (0, 1=w320:i16[])
              n372 = Build Array(w322) -> (w321:dbl[])
              n373 = To Double Precision Float(number=w320) -> (double precision float=w319:dbl[])
              n374 = Transpose 2D Array(2D array=w339) -> (transposed array=w338:dbl[][])
              n375 = Build Array (concatenate)(w321, w324, w323, w319, w296) -> (w345:dbl[])
              n376 = Insert Into Array(array=w338, new element=w345) -> (w341:dbl[][])  [unwired: 2 in]
              n377 = Transpose 2D Array(2D array=w341) -> (transposed array=w335:dbl[][])
              n378 = Array Size(array=w335) -> (size(s)=w334:i32[])
              n379 = Index Array(array=w334, index=1) -> (element=w333:i32)
              "size(s)" <- w333
              n380 = local read "stop Control General"() -> (w308:bool)
              n381 = local read "Program running"() -> (w312:bool)
              n382 = Quotient & Remainder(x=w344, y=599) -> (floor(x/y)=w340:i32)  [unwired: 1 out]
              n383 = local read "STOP ALL"() -> (w309:bool)
              n384 = local read "Guardando resumen"() -> (w294:bool)
              n385 = feedback-in #6(w340) -> ()
              n386 = feedback #6(w340) -> (w342:i32)
              n387 = Not Equal?(x=w340, y=w342) -> (x != y?=w313:bool)
              n388 = And(x=w313, y=w312) -> (x .and. y?=w293:bool)
              n389 = Or(x=w309, y=w308) -> (x .or. y?=w307:bool)
              n390 = Not(x=w294) -> (.not. x?=w292:bool)
              n391 = And(x=w292, y=w293) -> (x .and. y?=w291:bool)
              n392 = Or(x=w291, y=w307) -> (x .or. y?=w311:bool)
              "Guardando en disco" <- w311
              n393 = case shown="True" w311 {
                tunnel: w341 -> [w347 w350]
                tunnel: [w347 w352] -> w337
                tunnel: w333 -> [_ w349]
                tunnel: [dbl[][] [] w348] -> w305
                frame False {
                }
                frame True {
                  n394 = Delete From Array(array=w350, length=w349, index (row)=0) -> (deleted portion=w348:dbl[][], array with subset deleted=w352:dbl[][])  [unwired: 1 in]
                  "Guardar Array" <- w348
                }
              }
              "array w/ subset deleted" <- w337
              n395 = Transpose 2D Array(2D array=w305) -> (transposed array=w331:dbl[][])
              n396 = case shown="True" w311 {
                tunnel: string[] ["Time", "Segmento", "PWM1 (%)", "PWM2 (%)", "PWM3 (%)", "PWM4 (%)", "PWM5 (%)", "PWM6 (%)", "PWM7 (%)", "PWM8 (%)", "Setpoint T Peltier (ºC)", "T Valve 1 (ºC)", "T Valve 2 (ºC)", "T Valve 3 (ºC)", "T Valve 4 (ºC)", "T Valve 5 (ºC)", "T Valve 6 (ºC)", "T Valve 7 (ºC)", "T Valve 8 (ºC)", "Tª Bob V1 (ºC)", "Tª Bob V2 (ºC)", "Tª Bob V3 (ºC)", "Tª Bob V4 (ºC)", "Tª Bob V5 (ºC)", "Tª Bob V6 (ºC)", "Tª Bob V7 (ºC)", "Tª Bob V8 (ºC)", "HR RD CC (%)", "SP HR WR CC (%)", "T RD CC (ºC)", "SP T WR CC (ºC)", "Program Status", "Enable PI", "Entrada Bitron", "Run Program", "Pause", "Pause Entrar", "Stop control general", "DO H2 Lab", "Comunicación con PC"] -> [_ w365]
                tunnel: w331 -> [_ w364]
                tunnel: w327 -> [_ w363]
                tunnel: w307 -> [_ w362]
                tunnel: [FALSE ("STOP ALL") w361] -> w310
                frame False {
                }
                frame True {
                  n397 = flat-sequence {
                    tunnel: w365 -> [w371]
                    tunnel: w364 -> [w370]
                    tunnel: w363 -> [w369]
                    tunnel: w362 -> [w368]
                    tunnel: [w368] -> w360
                    tunnel: [w367] -> w357
                    tunnel: [w366] -> w355
                    tunnel: w360 -> [w389]
                    tunnel: [w389] -> w359
                    tunnel: [w385] -> w358
                    tunnel: w357 -> [w387]
                    tunnel: [w386] -> w356
                    tunnel: w355 -> [w388]
                    tunnel: [w404] -> w361
                    tunnel: w359 -> [w404]
                    tunnel: w358 -> [w403]
                    tunnel: w356 -> [w402]
                    tunnel: [FALSE ("reset warnings")] -> w354
                    frame #0 {
                      n398 = disable-structure shown="Disabled" {
                        frame Disabled {
                          n399 = call <vilib>:"Application Directory.vi"() -> ("Application Directory"=w377:path)
                          n400 = Build Path(base path=w377) -> (appended path=w376:path)  [unwired: 1 in]
                          n401 = Build Path(base path=w376, name or relative path=path "data CC.tdms") -> ()  [unwired: 1 out]
                        }
                        frame Enabled {
                        }
                      }
                      n402 = TDMS Open(10:T7."open or create" ("operation (0:open)"), 11:w369) -> (0:w373:errorcluster, 3:w374:refnum<k34>)  [unwired: 5 in]
                      n403 = TDMS Write(0:w374, 5:"Cámara climática" ("group name in (Untitled)"), 7:w371, 9:w370, 11:w373) -> (4:w366:refnum<k34>, 15:w367:errorcluster)  [unwired: 1 in, 2 out]
                      "Array" <- w370
                    }
                    frame #1 {
                      n404 = local read "Warnings table out"() -> (w382:T1)
                      n405 = for {
                        tunnel: w382 -> [w399] mode=indexing
                        shift-right: [w390] -> w380
                        shift-left: string[][] [] -> [w392]
                        n406 = Unbundle(w399) -> ("Time Stamp"=w397:timestamp, "Descripcion"=w393:string, "Numeric"=w396:i32)
                        n407 = Format Date/Time String(time format string (%c)="%<%.3X%x>T", seconds (now)=w397) -> (date/time string=w395:string)  [unwired: 1 in]
                        n408 = Number To Decimal String(number=w396) -> (decimal integer string=w394:string)  [unwired: 1 in]
                        n409 = Build Array(w395, w394, w393) -> (w391:string[])
                        n410 = Insert Into Array(array=w392, new element=w391) -> (w390:string[][])  [unwired: 2 in]
                      }
                      n411 = Transpose 2D Array(2D array=w380) -> (transposed array=w379:string[][])
                      n412 = TDMS Write(0:w388, 5:"Warnings/Errores" ("group name in (Untitled)"), 7:string[] ["Tiempo", "ID", "Descripción"] ("channel name(s) in (Untitled)"), 9:w379, 11:w387) -> (4:w386:refnum<k34>, 15:w385:errorcluster)  [unwired: 1 in, 2 out]
                    }
                    frame #2 {
                      n413 = TDMS Close(8:w403, 11:w402) -> ()  [unwired: 2 out]
                      n414 = local write "reset warnings"(TRUE ("reset warnings")) -> ()
                    }
                  }
                  n415 = local write "reset warnings"(w354) -> ()
                }
              }
              n416 = Transpose 2D Array(2D array=w337) -> (transposed array=w336:dbl[][])
              n417 = Wait Until Next ms Multiple(millisecond multiple=u32 10000 ("milliseconds to wait")) -> ()  [unwired: 1 out]
            }
            n418 = local write "stop Control General"(w281) -> ()
          }
        }
        n419 = local read "STOP ALL"() -> (w279:bool)
      }
      n420 = node-c288(w62) -> ()  [unwired: 1 out]
      n421 = node-c288(w36) -> ()  [unwired: 1 out]
      n422 = node-c288(w40) -> ()  [unwired: 1 out]
      n423 = call "Eurotherm_connect.vi"() -> ("error out"=w52:errorcluster, "Modbus Master out"=w53:refnum<class "Modbus Master.lvclass">)  [unwired: 10 in]
      n424 = node-c288() -> (w55:T4)  [unwired: 4 in]
      n425 = node-c288() -> (w57:T4)  [unwired: 4 in]
      n426 = timed-loop "Modbus Camara climatica" {
        timing: w55 -> [_]
        timing-out: [_] -> w54
        shift-right: [w876] -> w50
        shift-left: w53 -> [w880]
        shift-right: [w875] -> w51
        shift-left: w52 -> [w879]
        stop <- w864 stop-if-true
        n427 = node-c288() -> (→"Iteration Duration":i64)  [unwired: 1 in, 1 out]
        n428 = call "Eurotherm_read_TH.vi"("Modbus Master in"=w880, "error in (no error)"=w879) -> ("HR_rd"=w868:dbl, "Modbus Master out"=w878:refnum<class "Modbus Master.lvclass">, "Tª_rd"=→"Cam_Temp_read":dbl, "error out"=w877:errorcluster)  [unwired: 14 in]
        "Cam_Hum_read" <- w868
        n429 = local read "STOP ALL"() -> (w865:bool)
        n430 = Select(t=w868, s="Desconex_Control_Hum", f="Cam_Hum_write") -> (s? t:f=w870:dbl)
        n431 = case shown="False" w865 {
          selector: w865 -> [w881 w892]
          tunnel: w878 -> [w891 w902]
          tunnel: w877 -> [w887 w901]
          tunnel: [w889 w898] -> w876
          tunnel: [w888 w897] -> w875
          tunnel: "Cam_Write_Set_Temp" -> [_ w896]
          tunnel: "Cam_Temp_write" -> [_ w895]
          tunnel: "Cam_Write_Set_Hum" -> [_ w894]
          tunnel: w870 -> [_ w893]
          tunnel: [w881 w892] -> w864
          frame True {
            n432 = call "Eurotherm_write_T.vi"("error in (no error)"=w887, "Tª_sp"=25.0, "Tª write"=TRUE, "Modbus Master in"=w891) -> ("error out"=w886:errorcluster, "Modbus Master out"=w890:refnum<class "Modbus Master.lvclass">)  [unwired: 6 in]
            n433 = call "Eurotherm_write_H.vi"("error in (no error)"=w886, "HR_sp"=40.0, "HR write"=TRUE, "Modbus Master in"=w890) -> ("error out"=w888:errorcluster, "Modbus Master out"=w889:refnum<class "Modbus Master.lvclass">)  [unwired: 6 in]
          }
          frame False {
            n434 = call "Eurotherm_write_T.vi"("error in (no error)"=w901, "Tª_sp"=w895, "Tª write"=w896, "Modbus Master in"=w902) -> ("error out"=w899:errorcluster, "Modbus Master out"=w900:refnum<class "Modbus Master.lvclass">)  [unwired: 6 in]
            n435 = call "Eurotherm_write_H.vi"("error in (no error)"=w899, "HR_sp"=w893, "HR write"=w894, "Modbus Master in"=w900) -> ("error out"=w897:errorcluster, "Modbus Master out"=w898:refnum<class "Modbus Master.lvclass">)  [unwired: 6 in]
          }
        }
        n436 = node-c288() -> ()  [unwired: 1 in, 1 out]
      }
      n437 = timed-loop "Control Peltiers" {
        timing: w57 -> [_]
        timing-out: [_] -> w56
        stop <- w909 stop-if-true
        n438 = node-c288() -> ()  [unwired: 1 in, 1 out]
        n439 = case shown="False" "Disable PID" {
          frame True {
          }
          frame False {
            n440 = local read "Enable Test PID"() -> (w938:bool)
            n441 = Index Array(array="EnablePIs") -> (element #1=w937:bool, element #2=w936:bool, element #3=w935:bool, element #4=w934:bool, element #5=w933:bool, element #6=w932:bool, element #7=w931:bool, element #8=w930:bool)  [unwired: 8 in]
            n442 = case shown="True" w938 {
              tunnel: [w980 "Setpoint Peltiers"] -> w946
              tunnel: [w979 "Setpoint Peltiers"] -> w945
              tunnel: [w978 "Setpoint Peltiers"] -> w944
              tunnel: [w977 "Setpoint Peltiers"] -> w943
              tunnel: [w976 "Setpoint Peltiers"] -> w942
              tunnel: [w975 "Setpoint Peltiers"] -> w941
              tunnel: [w974 "Setpoint Peltiers"] -> w940
              tunnel: [w973 "Setpoint Peltiers"] -> w939
              frame True {
                n443 = local read "PID 1"() -> (w980:u32)
                n444 = local read "PID 2"() -> (w979:u32)
                n445 = local read "PID 3"() -> (w978:u32)
                n446 = local read "PID 4"() -> (w977:u32)
                n447 = local read "PID 5"() -> (w976:u32)
                n448 = local read "PID 6"() -> (w975:u32)
                n449 = local read "PID 7"() -> (w974:u32)
                n450 = local read "PID 8"() -> (w973:u32)
              }
              frame False {
              }
            }
            n451 = And(x="enable_PI", y=w937) -> (x .and. y?=w928:bool)
            n452 = And(x="enable_PI", y=w936) -> (x .and. y?=w927:bool)
            n453 = And(x="enable_PI", y=w935) -> (x .and. y?=w926:bool)
            n454 = And(x="enable_PI", y=w934) -> (x .and. y?=w925:bool)
            n455 = And(x="enable_PI", y=w933) -> (x .and. y?=w924:bool)
            n456 = And(x="enable_PI", y=w932) -> (x .and. y?=w923:bool)
            n457 = And(x="enable_PI", y=w931) -> (x .and. y?=w922:bool)
            n458 = And(x="enable_PI", y=w930) -> (x .and. y?=w921:bool)
            n459 = local read "T_valves"() -> (w918:dbl[])
            n460 = local read "T_valves"() -> (w956:dbl[])
            n461 = Index Array(array=w918, index #1=0 ("index")) -> (element #1=w917:dbl, element #2=w916:dbl, element #3=w915:dbl, element #4=w914:dbl, element #5=w913:dbl, element #6=w912:dbl, element #7=w911:dbl, element #8=w910:dbl)  [unwired: 7 in]
            n462 = Index Array(array=w956, index #1=8 ("index")) -> (element #1=w954:dbl, element #2=w953:dbl, element #3=w952:dbl, element #4=w951:dbl, element #5=w950:dbl, element #6=w949:dbl, element #7=w948:dbl, element #8=w947:dbl)  [unwired: 7 in]
            n463 = call "PI_valvulas.vi"("Temperatura manifold"=w917, "controlON"=w928, "Temperatura bobina"=w954, "Setpoint T"=w946) -> ("PWM (%)"=w969:dbl)  [unwired: 7 in]
            n464 = call "PI_valvulas5.vi"("Temperatura manifold"=w913, "controlON"=w924, "Temperatura bobina"=w950, "Setpoint T"=w942) -> ("PWM (%)"=w960:dbl)  [unwired: 7 in]
            n465 = To Unsigned Long Integer(number=w969) -> (unsigned 32bit integer=→"PWM 1 (%)":u32)
            n466 = To Unsigned Long Integer(number=w960) -> (unsigned 32bit integer=→"PWM 5 (%)":u32)
            n467 = call "PI_valvulas2.vi"("Temperatura manifold"=w916, "controlON"=w927, "Temperatura bobina"=w953, "Setpoint T"=w945) -> ("PWM (%)"=w972:dbl)  [unwired: 7 in]
            n468 = call "PI_valvulas6.vi"("Temperatura manifold"=w912, "controlON"=w923, "Temperatura bobina"=w949, "Setpoint T"=w941) -> ("PWM (%)"=w959:dbl)  [unwired: 7 in]
            n469 = To Unsigned Long Integer(number=w959) -> (unsigned 32bit integer=→"PWM 6 (%)":u32)
            n470 = To Unsigned Long Integer(number=w972) -> (unsigned 32bit integer=→"PWM 2 (%)":u32)
            n471 = call "PI_valvulas7.vi"("Temperatura manifold"=w911, "controlON"=w922, "Temperatura bobina"=w948, "Setpoint T"=w940) -> ("PWM (%)"=w958:dbl)  [unwired: 7 in]
            n472 = call "PI_valvulas3.vi"("Temperatura manifold"=w915, "controlON"=w926, "Temperatura bobina"=w952, "Setpoint T"=w944) -> ("PWM (%)"=w965:dbl)  [unwired: 7 in]
            n473 = To Unsigned Long Integer(number=w965) -> (unsigned 32bit integer=→"PWM 3 (%)":u32)
            n474 = To Unsigned Long Integer(number=w958) -> (unsigned 32bit integer=→"PWM 7 (%)":u32)
            n475 = call "PI_valvulas8.vi"("Temperatura manifold"=w910, "controlON"=w921, "Temperatura bobina"=w947, "Setpoint T"=w939) -> ("PWM (%)"=w957:dbl)  [unwired: 7 in]
            n476 = call "PI_valvulas4.vi"("Temperatura manifold"=w914, "controlON"=w925, "Temperatura bobina"=w951, "Setpoint T"=w943) -> ("PWM (%)"=w966:dbl)  [unwired: 7 in]
            n477 = To Unsigned Long Integer(number=w957) -> (unsigned 32bit integer=→"PWM 8 (%)":u32)
            n478 = To Unsigned Long Integer(number=w966) -> (unsigned 32bit integer=→"PWM 4 (%)":u32)
          }
        }
        n479 = local read "STOP ALL"() -> (w909:bool)
        n480 = node-c288() -> ()  [unwired: 1 in, 1 out]
      }
      n481 = node-c288() -> (w43:T4)  [unwired: 4 in]
      n482 = timed-loop "Simulación señal Bitron" {
        timing: w43 -> [_]
        timing-out: [_] -> w42
        stop <- w649 stop-if-true
        w648 = 0 ("FSM Bitron Simulacion")
        n483 = node-c288() -> ()  [unwired: 1 in, 1 out]
        n484 = local read "Run Program"() -> (w647:bool)
        n485 = And(x=w647, y="Activar Sim Bitron") -> (x .and. y?=w646:bool)
        n486 = case shown="True" w646 {
          tunnel: w648 -> [_ _]
          frame False {
          }
          frame True {
            n487 = disable-structure shown="Enabled" {
              frame Disabled {
                n488 = flat-sequence {
                  tunnel: [w659] -> w652
                  tunnel: w652 -> [w676]
                  frame #0 {
                    (unwired) 90.0 ("y")
                    w667 = u64 0 ("t")
                    n489 = First Call?() -> (First Call?: T/F=w672:bool)
                    n490 = case shown="True" w672 {
                      frame False {
                      }
                      frame True {
                        n491 = local write "Entrada digital Bitron"(FALSE ("Entrada digital Bitron")) -> ()
                      }
                    }
                    n492 = feedback #7(w667) -> (w665:u64)
                    n493 = Select(t=w667, s="Reset tempo", f=w665) -> (s? t:f=w654:u64)
                    "t ensayo (s)" <- w654
                    n494 = Increment(x=w654) -> (x+1=w666:u64)
                    n495 = feedback-in #7(w666) -> ()
                    n496 = To Double Precision Float(number=w654) -> (double precision float=w668:dbl)
                    n497 = Quotient & Remainder(x=w668, y=60.0) -> (x-y*floor(x/y)=→"segundos":dbl, floor(x/y)=w663:dbl)
                    "Minutos Totales" <- w663
                    n498 = Quotient & Remainder(x=w663, y="Minutos de medio ciclo") -> (floor(x/y)=w659:dbl)  [unwired: 1 out]
                    n499 = Quotient & Remainder(x=w663, y=60.0) -> (x-y*floor(x/y)=→"Minutos":dbl, floor(x/y)=w662:dbl)
                    n500 = Divide(x=w659, y=2.0) -> (x/y=→"Ciclos Totales":dbl)
                    n501 = Quotient & Remainder(x=w662, y=24.0) -> (x-y*floor(x/y)=→"Horas":dbl, floor(x/y)=→"días":dbl)
                  }
                  frame #1 {
                    n502 = feedback-in #8(w676) -> ()
                    n503 = feedback #8(w676) -> (w675:dbl)
                    n504 = Not Equal?(x=w676, y=w675) -> (x != y?=w674:bool)
                    n505 = case shown="True" w674 {
                      frame False {
                      }
                      frame True {
                        n506 = local read "Entrada digital Bitron"() -> (w677:bool)
                        n507 = Not(x=w677) -> (.not. x?=w678:bool)
                        n508 = local write "Entrada digital Bitron"(w678) -> ()
                      }
                    }
                  }
                }
              }
              frame Enabled {
                n509 = while {
                  stop <- w679 stop-if-true
                  n510 = Wait (ms)(milliseconds to wait=u32 500) -> ()  [unwired: 1 out]
                  n511 = local read "stop Control General"() -> (w681:bool)
                  n512 = local read "STOP ALL"() -> (w680:bool)
                  n513 = case shown="1" "FSM Bitron Simulacion" {
                    frame 1 {
                      n514 = flat-sequence {
                        frame #0 {
                          n515 = Tick Count (ms)() -> (millisecond timer value=w684:u32)
                          n516 = while {
                            tunnel: w684 -> [w694]
                            stop <- w688 stop-if-true
                            # "70 min  de ciclo"
                            n517 = Tick Count (ms)() -> (millisecond timer value=w695:u32)
                            n518 = Wait (ms)(milliseconds to wait=u32 500) -> ()  [unwired: 1 out]
                            n519 = Subtract(x=w695, y=w694) -> (x-y=w687:u32)
                            n520 = local read "stop Control General"() -> (w691:bool)
                            n521 = local read "STOP ALL"() -> (w692:bool)
                            n522 = Multiply(x=u32 60000 ("milliseconds to wait"), y="T cliclo (Bitron FSM Sim)") -> (x*y=w686:u32)
                            n523 = Greater Or Equal?(x=w687, y=w686) -> (x >= y?=w689:bool)
                            n524 = Or(x=w692, y=w691) -> (x .or. y?=w690:bool)
                            n525 = Or(x=w689, y=w690) -> (x .or. y?=w688:bool)
                          }
                        }
                        frame #1 {
                          n526 = local write "FSM Bitron Simulacion"(0 ("FSM Bitron Simulacion")) -> ()
                          n527 = local write "Entrada digital Bitron"(FALSE ("Entrada digital Bitron")) -> ()
                        }
                      }
                    }
                    frame 0, Default {
                      n528 = local read "DO H2 LAB"() -> (w699:bool)
                      n529 = case shown="True" w699 {
                        frame False {
                        }
                        frame True {
                          n530 = local write "FSM Bitron Simulacion"(1 ("FSM Bitron Simulacion")) -> ()
                          n531 = local write "Entrada digital Bitron"(TRUE ("Entrada digital Bitron")) -> ()
                        }
                      }
                    }
                  }
                  n532 = Or(x=w680, y=w681) -> (x .or. y?=w679:bool)
                }
              }
            }
          }
        }
        n533 = local write "FSM Bitron Simulacion"(w648) -> ()
        n534 = local read "STOP ALL"() -> (w649:bool)
        n535 = node-c288() -> ()  [unwired: 1 in, 1 out]
      }
      n536 = node-c288() -> (w49:T4)  [unwired: 4 in]
      n537 = timed-loop "FSM Control" {
        timing: w49 -> [_]
        timing-out: [_] -> w48
        stop <- w707 stop-if-true
        w706 = FALSE ("Pausa")
        w708 = u16 0 ("Segmento_temp")
        # "Reset Variables locales"
        # "Condiciones inicales T ambiente"
        n538 = node-c288() -> ()  [unwired: 1 in, 1 out]
        n539 = local write "Cam_Write_Set_Temp"(TRUE ("Enable_Temp_write")) -> ()
        n540 = local write "Cam_Temp_write"(25.0 ("Setpoint_temp_write")) -> ()
        n541 = local write "DO H2 LAB"(FALSE ("DO H2 LAB")) -> ()
        n542 = local write "Pausa entrar"(w706) -> ()
        n543 = local write "Segmento"(w708) -> ()
        n544 = local write "enable_PI"(w706) -> ()
        n545 = local write "Pausa"(w706) -> ()
        n546 = case shown="True" "Run Program" {
          tunnel: w708 -> [_ _]
          tunnel: w706 -> [_ _]
          frame False {
          }
          frame True {
            # "Main"
            n547 = while {
              tunnel: [FALSE ("Run Program")] -> w712
              stop <- w714 stop-if-true
              # "0 -> First Time. Frío hasta -30 y señal bitron\n1 -> Transitorio frio\n2 -> Estabilidad frio\n3 -> Transitorio calor\n4 -> Estabilidad calor"
              # "Para el primer ciclo, detectamos el flanco de Run Program\ny almacenamos el tiempo incial.\nPara el resto de ciclos, detectamos que haya habido un cambio\nde segmento y que el actual sea 4 (Cuando empieza a enfriar)."
              n548 = local write "Program running"(TRUE ("Program running")) -> ()
              n549 = Select(t=u16 50, s="Pausa", f="Segmento") -> (s? t:f=w720:u16)
              n550 = Select(t=u16 20, s="Enable Test PID", f=w720) -> (s? t:f=w717:u16)
              "Segmento act" <- w717
              n551 = case shown="0, Default" w717 {
                tunnel: "Setpoint Frío" -> [w746 w757 _ _ _ _ _]
                tunnel: "Setpoint Corte Frío" -> [w744 w756 w787 _ _ _ _]
                frame 0, Default {
                  n552 = local write "Cam_Write_Set_Temp"(TRUE ("Enable_Temp_write")) -> ()
                  n553 = local write "Setpoint Peltiers"(w746) -> ()
                  n554 = local write "Cam_Temp_write"(w746) -> ()
                  n555 = local write "Cam_Hum_write"(0.0 ("Cam_Hum_write")) -> ()
                  n556 = local write "Rampa_pelt"(FALSE ("Rampa_cam")) -> ()
                  n557 = local write "Rampa_cam"(FALSE ("Rampa_cam")) -> ()
                  n558 = local write "enable_PI"(FALSE ("Enable_PI")) -> ()
                  n559 = local write "Cam_Write_Set_Hum"(TRUE ("Cam_Write_Set_Hum")) -> ()
                  n560 = local read "mean_T_valves"() -> (w740:dbl)
                  n561 = local read "Entrada digital Bitron"() -> (w742:bool)
                  n562 = local read "DO H2 LAB"() -> (w743:bool)
                  n563 = Less Or Equal?(x=w740, y=w744) -> (x <= y?=w745:bool)
                  n564 = And(x=w743, y=w742) -> (x .and. y?=w741:bool)
                  n565 = case shown="True" w741 {
                    frame False {
                    }
                    frame True {
                      n566 = Tick Count (ms)() -> (millisecond timer value=w750:u32)
                      n567 = local write "Timer 3 (Inicio Transitorio Calor)"(w750) -> ()
                      n568 = local write "Segmento"(u16 3 ("Segmento_temp")) -> ()
                    }
                  }
                  n569 = case shown="True" w745 {
                    frame False {
                    }
                    frame True {
                      n570 = local write "DO H2 LAB"(TRUE ("DO H2 LAB")) -> ()
                    }
                  }
                }
                frame 1 {
                  # "Segmento escalon frío"
                  # "(Luego -38)"
                  # "(para debuggar -5)"
                  # "(Ahora para debuggar ponemos T amb)"
                  # "Segmento -40"
                  n571 = local write "Cam_Write_Set_Temp"(TRUE ("Enable_Temp_write")) -> ()
                  n572 = local write "Setpoint Peltiers"(w757) -> ()
                  n573 = local write "Cam_Temp_write"(w757) -> ()
                  n574 = local write "Cam_Write_Set_Hum"(TRUE ("Cam_Write_Set_Hum")) -> ()
                  n575 = local write "Cam_Hum_write"(0.0 ("Cam_Hum_write")) -> ()
                  n576 = local read "mean_T_valves"() -> (w753:dbl)
                  n577 = Add(x=w756, y=2.0) -> (x+y=w754:dbl)
                  n578 = Less Or Equal?(x=w753, y=w754) -> (x <= y?=w761:bool)
                  n579 = case shown="True" w761 {
                    frame False {
                      n580 = local write "enable_PI"(FALSE ("Enable_PI")) -> ()
                    }
                    frame True {
                      n581 = Tick Count (ms)() -> (millisecond timer value=→"Timer 2 (Inicio Estabilidad Frio)":u32)
                      n582 = local write "Segmento"(u16 2 ("Segmento_temp")) -> ()
                    }
                  }
                }
                frame 2 {
                  # "90 min en ms"
                  # "15 min en ms"
                  # "100 min en ms"
                  # "Segmento estabilidad frío"
                  # "Ponemos un boton para debugar"
                  # "Esperar a lectura digital"
                  # "Activar salida digital"
                  n583 = local write "Setpoint Peltiers"(w787) -> ()
                  n584 = local write "Cam_Temp_write"(w787) -> ()
                  n585 = local write "Cam_Write_Set_Temp"(TRUE ("Cam_Write_Set_Temp")) -> ()
                  n586 = local write "Cam_Write_Set_Hum"(FALSE ("Cam_Write_Set_Hum")) -> ()
                  n587 = Tick Count (ms)() -> (millisecond timer value=w781:u32)
                  n588 = local read "Timer 2 (Inicio Estabilidad Frio)"() -> (w778:u32)
                  n589 = local read "Timer 1 (Inicio transitorio frio)"() -> (w780:u32)
                  n590 = Subtract(x=w781, y=w778) -> (x-y=w779:u32)
                  n591 = Subtract(x=w781, y=w780) -> (x-y=w782:u32)
                  n592 = local read "DO H2 LAB"() -> (w767:bool)
                  n593 = Multiply(x=u32 60000, y="Tiempo minimo de ciclo") -> (x*y=w773:u32)
                  n594 = Less?(x=w782, y=w773) -> (x < y?=w785:bool)
                  n595 = Multiply(x=u32 60000, y="Tiempò en estabilidad de Frío") -> (x*y=w777:u32)
                  n596 = Greater Or Equal?(x=w779, y=w777) -> (x >= y?=w784:bool)
                  n597 = And(x="Entrada digital Bitron", y=w767) -> (x .and. y?=w765:bool)
                  n598 = Multiply(x=u32 60000, y="Tiempo maximo de ciclo") -> (x*y=w769:u32)
                  n599 = Greater Or Equal?(x=w782, y=w769) -> (x >= y?=w783:bool)
                  n600 = And(x=w785, y=w784) -> (x .and. y?=w786:bool)
                  n601 = Or(x=w783, y=w786) -> (x .or. y?=w768:bool)
                  n602 = case shown="True" w765 {
                    frame False {
                    }
                    frame True {
                      n603 = Tick Count (ms)() -> (millisecond timer value=→"Timer 3 (Inicio Transitorio Calor)":u32)
                      n604 = local write "Segmento"(u16 3 ("Segmento_temp")) -> ()
                    }
                  }
                  n605 = case shown="True" w768 {
                    frame False {
                    }
                    frame True {
                      n606 = local write "DO H2 LAB"(TRUE ("DO H2 LAB")) -> ()
                    }
                  }
                }
                frame 3 {
                  # "Segmento rampa calor"
                  # "Rampa camara climatica"
                  # "Habilitamos rampa PI desde -40"
                  # "estaba a40_ Igual interesaría bajar la humedad a 10 %"
                  n607 = local write "Cam_Write_Set_Temp"(TRUE ("Enable_Temp_write")) -> ()
                  n608 = local write "Rampa_pelt"(TRUE ("Rampa_cam")) -> ()
                  n609 = local write "Rampa_cam"(TRUE ("Rampa_cam")) -> ()
                  n610 = local write "enable_PI"(TRUE ("Enable_PI")) -> ()
                  n611 = local write "Cam_Write_Set_Hum"(TRUE ("Cam_Write_Set_Hum")) -> ()
                  n612 = local write "Cam_Hum_write"(10.0 ("Cam_Hum_write")) -> ()
                  n613 = local read "Setpoint calor cam"() -> (w800:dbl)
                  n614 = local read "Entrada digital Bitron"() -> (w794:bool)
                  n615 = local read "Cam_Temp_read"() -> (w797:dbl)
                  n616 = Subtract(x=w800, y=5.0) -> (x-y=w798:dbl)
                  n617 = Not(x=w794) -> (.not. x?=w793:bool)
                  n618 = Greater Or Equal?(x=w797, y=w798) -> (x >= y?=w796:bool)
                  n619 = Or(x=w796, y=w793) -> (x .or. y?=w795:bool)
                  n620 = case shown="True" w795 {
                    frame False {
                    }
                    frame True {
                      n621 = Tick Count (ms)() -> (millisecond timer value=→"Timer 4 (Inicio Estabilidad Calor)":u32)
                      n622 = local write "Segmento"(u16 4 ("Segmento_temp")) -> ()
                    }
                  }
                }
                frame 4 {
                  # "Segmento estabilidad calor"
                  # "Ponemos un boton para debugar"
                  # "Esperar a lectura digital"
                  n623 = local write "Cam_Write_Set_Hum"(FALSE ("Cam_Write_Set_Hum")) -> ()
                  n624 = local write "Cam_Write_Set_Temp"(FALSE ("Enable_Temp_write")) -> ()
                  n625 = local read "Entrada digital Bitron"() -> (w809:bool)
                  n626 = case shown="False" w809 {
                    frame False {
                      n627 = Tick Count (ms)() -> (millisecond timer value=→"Timer 1 (Inicio transitorio frio)":u32)
                      n628 = local write "DO H2 LAB"(FALSE ("DO H2 LAB")) -> ()
                      n629 = local write "Segmento"(u16 1 ("Segmento_temp")) -> ()
                    }
                    frame True {
                    }
                  }
                }
                frame 20 {
                  w825 = FALSE ("enable_PI")
                  n630 = local write "Rampa_pelt"(w825) -> ()
                  n631 = local write "Rampa_cam"(w825) -> ()
                  n632 = local write "enable_PI"(TRUE ("Rampa_pelt")) -> ()
                  n633 = Index Array(array="Test PID") -> (element #1=→"PID 1":u32, element #2=→"PID 2":u32, element #3=→"PID 3":u32, element #4=→"PID 4":u32, element #5=→"PID 5":u32, element #6=→"PID 6":u32, element #7=→"PID 7":u32, element #8=→"PID 8":u32)  [unwired: 8 in]
                }
                frame 50 {
                  n634 = local write "Cam_Write_Set_Temp"(FALSE ("Cam_Write_Set_Temp")) -> ()
                  n635 = case shown="True" "Pausa entrar" {
                    frame False {
                    }
                    frame True {
                      n636 = local read "Cam_Temp_write"() -> (w837:dbl)
                      n637 = local read "Rampa_pelt"() -> (w830:bool)
                      n638 = flat-sequence {
                        tunnel: w837 -> [w846]
                        tunnel: [w846] -> w839
                        tunnel: w836 -> [w842]
                        tunnel: [w842] -> w835
                        tunnel: [w841] -> w832
                        tunnel: w831 -> [w841]
                        tunnel: w830 -> [w840]
                        tunnel: [w840] -> w829
                        tunnel: w839 -> [w850]
                        tunnel: [w850] -> w838
                        tunnel: w835 -> [w849]
                        tunnel: [w849] -> w834
                        tunnel: [w848] -> w833
                        tunnel: w832 -> [w848]
                        tunnel: w829 -> [w847]
                        tunnel: [w847] -> w828
                        tunnel: w838 -> [w858]
                        tunnel: w834 -> [w856]
                        tunnel: w833 -> [w855]
                        tunnel: w828 -> [w854]
                        frame #0 {
                          w843 = FALSE ("Enable_PI")
                          n639 = local write "Cam_Write_Set_Temp"(TRUE ("Cam_Write_Set_Temp")) -> ()
                          n640 = local write "Cam_Temp_write"(25.0 ("Setpoint_temp_write")) -> ()
                          n641 = local write "enable_PI"(w843) -> ()
                          n642 = local write "enable_PI"(w843) -> ()
                          n643 = local write "Rampa_pelt"(w843) -> ()
                        }
                        frame #1 {
                          n644 = while {
                            stop <- w853 stop-if-true
                            n645 = local read "Pausa entrar"() -> (w852:bool)
                            n646 = Wait (ms)(milliseconds to wait=u32 200) -> ()  [unwired: 1 out]
                            n647 = Not(x=w852) -> (.not. x?=w853:bool)
                          }
                        }
                        frame #2 {
                          n648 = local write "Rampa_pelt"(w854) -> ()
                          n649 = local write "Cam_Temp_write"(w858) -> ()
                          n650 = local write "enable_PI"(w855) -> ()
                          n651 = local write "enable_PI"(w856) -> ()
                          n652 = local write "Cam_Write_Set_Temp"(TRUE ("Cam_Write_Set_Temp")) -> ()
                        }
                        frame #3 {
                          n653 = Wait (ms)(milliseconds to wait=u32 500) -> ()  [unwired: 1 out]
                        }
                      }
                      n654 = local read "enable_PI"() -> (w831:bool)
                      n655 = local read "enable_PI"() -> (w836:bool)
                    }
                  }
                }
              }
              n656 = local read "Enable Test PID"() -> (w713:bool)
              n657 = case shown="False" w713 {
                frame False {
                  n658 = local write "Disable PID"(FALSE ("Disable PID")) -> ()
                  n659 = property on="Disable PID" class="Bool (strict)"("DisabledEnum"=T3."Disabled" ("Disabled")) -> ()  [unwired: 2 in, 2 out]
                }
                frame True {
                  n660 = property on="Disable PID" class="Bool (strict)"("DisabledEnum"=T3."Enabled" ("Disabled")) -> ()  [unwired: 2 in, 2 out]
                }
              }
              n661 = local read "STOP ALL"() -> (w724:bool)
              n662 = Or(x=w724, y="stop Control General") -> (x .or. y?=w715:bool)
              n663 = case shown="True" w715 {
                selector: w715 -> [_ w735]
                tunnel: [FALSE w735] -> w714
                frame False {
                }
                frame True {
                  w736 = u32 0 ("PWM 1 (%)")
                  n664 = local write "Disable PID"(FALSE ("Disable PID")) -> ()
                  n665 = local write "PWM 8 (%)"(w736) -> ()
                  n666 = local write "PWM 6 (%)"(w736) -> ()
                  n667 = local write "PWM 7 (%)"(w736) -> ()
                  n668 = local write "PWM 5 (%)"(w736) -> ()
                  n669 = local write "PWM 4 (%)"(w736) -> ()
                  n670 = local write "PWM 1 (%)"(w736) -> ()
                  n671 = local write "PWM 2 (%)"(w736) -> ()
                  n672 = local write "PWM 3 (%)"(w736) -> ()
                }
              }
              n673 = Wait (ms)(milliseconds to wait=u32 200) -> ()  [unwired: 1 out]
            }
            n674 = local write "Run Program"(w712) -> ()
          }
        }
        n675 = local read "STOP ALL"() -> (w707:bool)
        n676 = node-c288() -> ()  [unwired: 1 in, 1 out]
        "Program running" <- w706
        "First Time" <- TRUE
      }
      n677 = node-c288(w54) -> ()  [unwired: 1 out]
      n678 = node-c288(w56) -> ()  [unwired: 1 out]
      n679 = node-c288(w42) -> ()  [unwired: 1 out]
      n680 = node-c288(w48) -> ()  [unwired: 1 out]
    }
    frame #2 {
      w1033 = u32 0 ("PWM_DO0")
      # "End"
      n681 = call-dynamic "Close.vi"("error in (no error)"=w1031, "Modbus master in"=w1032) -> ("error out"=w1030:errorcluster)  [unwired: 9 in]
      n682 = call-dynamic "Close.vi"("error in (no error)"=w1045, "Modbus master in"=w1044) -> ("error out"=w1042:errorcluster)  [unwired: 9 in]
      n683 = local write "STOP ALL"(FALSE ("stop")) -> ()
      n684 = local write "PWM 8 (%)"(w1033) -> ()
      n685 = local write "PWM 6 (%)"(w1033) -> ()
      n686 = local write "PWM 7 (%)"(w1033) -> ()
      n687 = local write "PWM 5 (%)"(w1033) -> ()
      n688 = local write "PWM 4 (%)"(w1033) -> ()
      n689 = local write "PWM 1 (%)"(w1033) -> ()
      n690 = local write "PWM 2 (%)"(w1033) -> ()
      n691 = xnode "Read/Write Control"("FPGA VI Reference In"=w1037, "error in"=w1036) -> ("FPGA VI Reference Out"=w1035:refnum<k20>, "error out"=w1034:errorcluster)  [unwired: 8 in]
      n692 = local write "PWM 3 (%)"(w1033) -> ()
      n693 = call <vilib>:"DAQmx Stop Task.vi"("task/channels in"=w1040, "error in"=w1039) -> ("error out"=w1038:errorcluster)  [unwired: 12 in, 1 out]
      n694 = xnode "Close FPGA VI Reference"("FPGA VI Reference In"=w1035, "error in"=w1034) -> ("error out"=w1041:errorcluster)
      n695 = Merge Errors(w1038, w1041, w1042, w1030) -> (w1043:errorcluster)
      n696 = call <vilib>:"Simple Error Handler.vi"("error in (no error)"=w1043) -> ()  [unwired: 4 in, 5 out]
    }
  }
